vi "TestExecutive V2.vi"() -> ()   [LabVIEW 2025]
uses:
  controls/TestDefinition.ctl
  controls/SingleTest.ctl
  controls/TestType.ctl
  controls/HTR Test Options.ctl
  controls/TestFailOptions.ctl
  controls/TED4015 Status.ctl
  controls/Diode Test Options.ctl
  <vilib>/addons/_JKI Toolkits/State Machine/_JKI_lib_State_Machine.llb/Periodic Trigger__ogtk__JKI-SM__jki_lib_state_machine.vi
  <vilib>/addons/_JKI Toolkits/State Machine/_JKI_lib_State_Machine.llb/Select State(s)_err__jki_lib_state_machine.vi
  <userlib>/_OpenG.lib/time/time.llb/openg_time.lvlib
panel:
  in  "Exit":bool
  out "Camera":string="HD Pro Webcam C920"
  out "TopFolderPath":path=path "d:/LTM Tests/MechanismLTM/HeaterTest_25-11-11_16-31-07"
  out "TopFolderPrefix":string="HeaterTest_25-11-11_16-31-07"
  out "Status":string="Setup - Fill in fields and press Next to Continue"
  in  "Main Tabs":T1(tab)
  in  "Cycles To Run":i32=1 min=1 max=200
  in  "Next1":bool
  in  "Loggers Directory":path=path "d:/LTM Tests/MechanismLTM"
  in  "Test Name":string="HeaterTest"
  in  "FFMPEG exe":path=path "C:/Program Files/FFMpeg/bin/ffmpeg.exe"
  in  "Path to Actuation Script":path=path "C:/Users/dpl/Documents/ob_egse/src/main.py"
  in  "StartCycle":i32
  in  "Tab Control":T2(tab)=enum."Diodes"
  in  "TVC_Temperatures":waveform(dbl)[](array[waveform])=[{"t0"=timestamp(3820413812.1049423 s since 1904-01-01), "dt"=1.0, "Y"=[-45.0], "attributes"=variant("NI_ChannelName"=variant(string "3A"))}, {"t0"=timestamp(3820413812.1049423 s since 1904-01-01), "dt"=1.0, "Y"=[0.1969585335155295], "attributes"=variant("NI_ChannelName"=variant(string "3B"))}, {"t0"=timestamp(3820413812.1049423 s since 1904-01-01), "dt"=1.0, "Y"=[0.2898606356704896], "attributes"=variant("NI_ChannelName"=variant(string "3C"))}, {"t0"=timestamp(3820413812.1049423 s since 1904-01-01), "dt"=1.0, "Y"=[0.3274623555028864], "attributes"=variant("NI_ChannelName"=variant(string "3D"))}, {"t0"=timestamp(3820413812.1049423 s since 1904-01-01), "dt"=1.0, "Y"=[0.3794250746071903], "attributes"=variant("NI_ChannelName"=variant(string "4A"))}, {"t0"=timestamp(3820413812.1049423 s since 1904-01-01), "dt"=1.0, "Y"=[0.7650917242886434], "attributes"=variant("NI_ChannelName"=variant(string "4B"))}, {"t0"=timestamp(3820413812.1049423 s since 1904-01-01), "dt"=1.0, "Y"=[0.4416685188806395], "attributes"=variant("NI_ChannelName"=variant(string "4C"))}, {"t0"=timestamp(3820413812.1049423 s since 1904-01-01), "dt"=1.0, "Y"=[0.7497510727682433], "attributes"=variant("NI_ChannelName"=variant(string "4D"))}, {"t0"=timestamp(3820413812.1049423 s since 1904-01-01), "dt"=1.0, "Y"=[0.8015992709050663], "attributes"=variant("NI_ChannelName"=variant(string "Target"))}]
  out "ChannelNames":string[](array[string])=["3A", "3B", "3C", "3D", "4A", "4B", "4C", "4D", "Target"]
  in  "ControlChannel":u16(ring) items=["3A", "3B", "3C", "3D", "4A", "4B", "4C", "4D", "Target"]
  in  "TLUP_Temperatures":waveform(dbl)[](array[waveform])=[{"t0"=timestamp(3820413812.102944 s since 1904-01-01), "dt"=1.0, "Y"=[23.56152], "attributes"=variant("NI_ChannelName"=variant(string "TLUP_0"))}, {"t0"=timestamp(3820413812.102944 s since 1904-01-01), "dt"=1.0, "Y"=[-999.0], "attributes"=variant("NI_ChannelName"=variant(string "TLUP_1"))}, {"t0"=timestamp(3820413812.102944 s since 1904-01-01), "dt"=1.0, "Y"=[-999.0], "attributes"=variant("NI_ChannelName"=variant(string "TLUP_2"))}, {"t0"=timestamp(3820413812.102944 s since 1904-01-01), "dt"=1.0, "Y"=[-999.0], "attributes"=variant("NI_ChannelName"=variant(string "TLUP_3"))}, {"t0"=timestamp(3820413812.102944 s since 1904-01-01), "dt"=1.0, "Y"=[nan], "attributes"=variant("NI_ChannelName"=variant(string "TLUP_4"))}, {"t0"=timestamp(3820413812.102944 s since 1904-01-01), "dt"=1.0, "Y"=[nan], "attributes"=variant("NI_ChannelName"=variant(string "TLUP_5"))}, {"t0"=timestamp(3820413812.102944 s since 1904-01-01), "dt"=1.0, "Y"=[nan], "attributes"=variant("NI_ChannelName"=variant(string "TLUP_6"))}, {"t0"=timestamp(3820413812.102944 s since 1904-01-01), "dt"=1.0, "Y"=[nan], "attributes"=variant("NI_ChannelName"=variant(string "TLUP_7"))}]
  in  "PSU_Monitor":waveform(dbl)[](array[waveform])=[{"t0"=timestamp(3820413812.1099424 s since 1904-01-01), "dt"=1.0, "Y"=[2.52], "attributes"=variant("NI_ChannelName"=variant(string "Board_Voltage_0"))}, {"t0"=timestamp(3820413812.1153584 s since 1904-01-01), "dt"=1.0, "Y"=[-0.009], "attributes"=variant("NI_ChannelName"=variant(string "Board_Voltage_0"))}, {"t0"=timestamp(3820413812.1099424 s since 1904-01-01), "dt"=1.0, "Y"=[-0.017], "attributes"=variant("NI_ChannelName"=variant(string "Board_Current_0"))}, {"t0"=timestamp(3820413812.1153584 s since 1904-01-01), "dt"=1.0, "Y"=[0.0], "attributes"=variant("NI_ChannelName"=variant(string "Board_Current_0"))}]
  in  "PSU Enable":bool
  in  "Heater Monitor":waveform(dbl)[](array[waveform])=[{"t0"=timestamp(3820413812.092942 s since 1904-01-01), "dt"=1.0, "Y"=[-0.005], "attributes"=variant("NI_ChannelName"=variant(string "Heater_Voltage"))}, {"t0"=timestamp(3820413812.092942 s since 1904-01-01), "dt"=1.0, "Y"=[1.55], "attributes"=variant("NI_ChannelName"=variant(string "Heater_Current"))}]
  in  "Heater Enable":bool
  in  "COM Port":i32=21 min=1 max=63 step=1
  in  "Video Camera":u16(ring) items=["USB Camera"]
  in  "TED":waveform(dbl)[](graph)
  in  "TEC On":bool[](array[boolean])=[FALSE, FALSE]
  in  "TED Status":T3[](array[typedef])=[{"Output"=TRUE, "SetPoint"=0.0, "Temperature"=0.0, "Current"=0.0, "Voltage"=0.0, "CableTrip"=FALSE, "TransducerTrip"=FALSE, "OverTemp"=FALSE}, {"Output"=TRUE, "SetPoint"=0.0, "Temperature"=0.0, "Current"=0.0, "Voltage"=0.0, "CableTrip"=FALSE, "TransducerTrip"=FALSE, "OverTemp"=FALSE}]
  in  "LED_Stimulate":bool
  in  "LED_Illuminate":bool
  in  "Diode Currents":waveform(dbl)[](graph)=[{"t0"=timestamp(0 s since 1904-01-01), "dt"=1.0, "Y"=[2.0]}, {"t0"=timestamp(0 s since 1904-01-01), "dt"=1.0, "Y"=[2.0]}]
  in  "Next2":bool
  in  "Server IP":u16(ring) items=["localhost", "172.17.52.10"]
  in  "SaveTests":bool
  in  "TestDefinition":T4={"Tests"=[{"TTrigger"=-130.0, "Direction"=enum."Falling", "TDelay"=0.0, "Type"=enum."No Test", "Pre-Log (s)"=0.0, "Duration (s)"=0.0, "Post-Log(s)"=0.0}, {"TTrigger"=-80.0, "Direction"=enum."Rising", "TDelay"=0.0, "Type"=enum."Heater Test", "Pre-Log (s)"=10.0, "Duration (s)"=10.0, "Post-Log(s)"=2.0}, {"TTrigger"=-50.0, "Direction"=enum."Rising", "TDelay"=0.0, "Type"=enum."Diode Test", "Pre-Log (s)"=20.0, "Duration (s)"=20.0, "Post-Log(s)"=20.0}, {"TTrigger"=-45.0, "Direction"=enum."Rising", "TDelay"=0.0, "Type"=enum."Actuation Test", "Pre-Log (s)"=10.0, "Duration (s)"=20.0, "Post-Log(s)"=10.0}, {"TTrigger"=30.0, "Direction"=enum."Rising", "TDelay"=0.0, "Type"=enum."Actuation Test", "Pre-Log (s)"=10.0, "Duration (s)"=30.0, "Post-Log(s)"=100.0}, {"TTrigger"=40.0, "Direction"=enum."Rising", "TDelay"=30.0, "Type"=enum."No Test", "Pre-Log (s)"=10.0, "Duration (s)"=30.0, "Post-Log(s)"=100.0}], "ActuationsPerLoop"=2, "Temperature Log Period(ms)"=1000, "PSU  Log Period (ms)"=100} {"Tests"."Post-Log(s)" format="%#_13g"; "Tests"."Pre-Log (s)" format="%#_13g"; "Tests"."Duration (s)" format="%#_13g"}
  in  "Next Button 3":bool
  in  "Heater Test Options":T7={"Heater Nominal Current (A)"=0.67, "Heater Current Tolerance (%)"=20.0, "Fail Text"="", "Fail Option"=enum."Ignore"} {"Heater Current Tolerance (%)" min=1.0 max=100.0; "Heater Nominal Current (A)" min=0.0 max=1.0}
  in  "Diode Test Options":T9={"Temp.Tol"=0.1, "Max IDark"=[], "Min ILight"=[0.1, 1e-08]}
  out "Messages":string
  out "ACT Fault":bool
  out "TVC_StopAfterCycle":bool
  out "Diode Logging":bool
  out "Master Logging":bool
  out "DelayRemaining":string
  out "HTR On":bool
  out "Temperatures":dynamicdata(graph)=[{"t0"=timestamp(3820413812.1049423 s since 1904-01-01), "dt"=1.0, "Y"=[-45.0], "attributes"=variant("NI_ChannelName"=variant(string "3A"))}, {"t0"=timestamp(3820413812.1049423 s since 1904-01-01), "dt"=1.0, "Y"=[0.1969585335155295], "attributes"=variant("NI_ChannelName"=variant(string "3B"))}, {"t0"=timestamp(3820413812.1049423 s since 1904-01-01), "dt"=1.0, "Y"=[0.2898606356704896], "attributes"=variant("NI_ChannelName"=variant(string "3C"))}, {"t0"=timestamp(3820413812.1049423 s since 1904-01-01), "dt"=1.0, "Y"=[0.3274623555028864], "attributes"=variant("NI_ChannelName"=variant(string "3D"))}, {"t0"=timestamp(3820413812.1049423 s since 1904-01-01), "dt"=1.0, "Y"=[0.3794250746071903], "attributes"=variant("NI_ChannelName"=variant(string "4A"))}, {"t0"=timestamp(3820413812.1049423 s since 1904-01-01), "dt"=1.0, "Y"=[0.7650917242886434], "attributes"=variant("NI_ChannelName"=variant(string "4B"))}, {"t0"=timestamp(3820413812.1049423 s since 1904-01-01), "dt"=1.0, "Y"=[0.4416685188806395], "attributes"=variant("NI_ChannelName"=variant(string "4C"))}, {"t0"=timestamp(3820413812.1049423 s since 1904-01-01), "dt"=1.0, "Y"=[0.7497510727682433], "attributes"=variant("NI_ChannelName"=variant(string "4D"))}, {"t0"=timestamp(3820413812.1049423 s since 1904-01-01), "dt"=1.0, "Y"=[0.8015992709050663], "attributes"=variant("NI_ChannelName"=variant(string "Target"))}, {"t0"=timestamp(3820413812.102944 s since 1904-01-01), "dt"=1.0, "Y"=[23.56152], "attributes"=variant("NI_ChannelName"=variant(string "TLUP_0"))}, {"t0"=timestamp(3820413812.102944 s since 1904-01-01), "dt"=1.0, "Y"=[-999.0], "attributes"=variant("NI_ChannelName"=variant(string "TLUP_1"))}, {"t0"=timestamp(3820413812.102944 s since 1904-01-01), "dt"=1.0, "Y"=[-999.0], "attributes"=variant("NI_ChannelName"=variant(string "TLUP_2"))}, {"t0"=timestamp(3820413812.102944 s since 1904-01-01), "dt"=1.0, "Y"=[-999.0], "attributes"=variant("NI_ChannelName"=variant(string "TLUP_3"))}, {"t0"=timestamp(3820413812.102944 s since 1904-01-01), "dt"=1.0, "Y"=[nan], "attributes"=variant("NI_ChannelName"=variant(string "TLUP_4"))}, {"t0"=timestamp(3820413812.102944 s since 1904-01-01), "dt"=1.0, "Y"=[nan], "attributes"=variant("NI_ChannelName"=variant(string "TLUP_5"))}, {"t0"=timestamp(3820413812.102944 s since 1904-01-01), "dt"=1.0, "Y"=[nan], "attributes"=variant("NI_ChannelName"=variant(string "TLUP_6"))}, {"t0"=timestamp(3820413812.102944 s since 1904-01-01), "dt"=1.0, "Y"=[nan], "attributes"=variant("NI_ChannelName"=variant(string "TLUP_7"))}]
  out "Trigger Point Reading":dbl=-45.0
  out "ACT Logging":bool
  out "HTR Log":bool
  out "TVC_CyclesRemaining":i32
  in  "TVC_CycleNumber":i32
  out "HTR_Fault":bool
  out "TEC Fault":bool
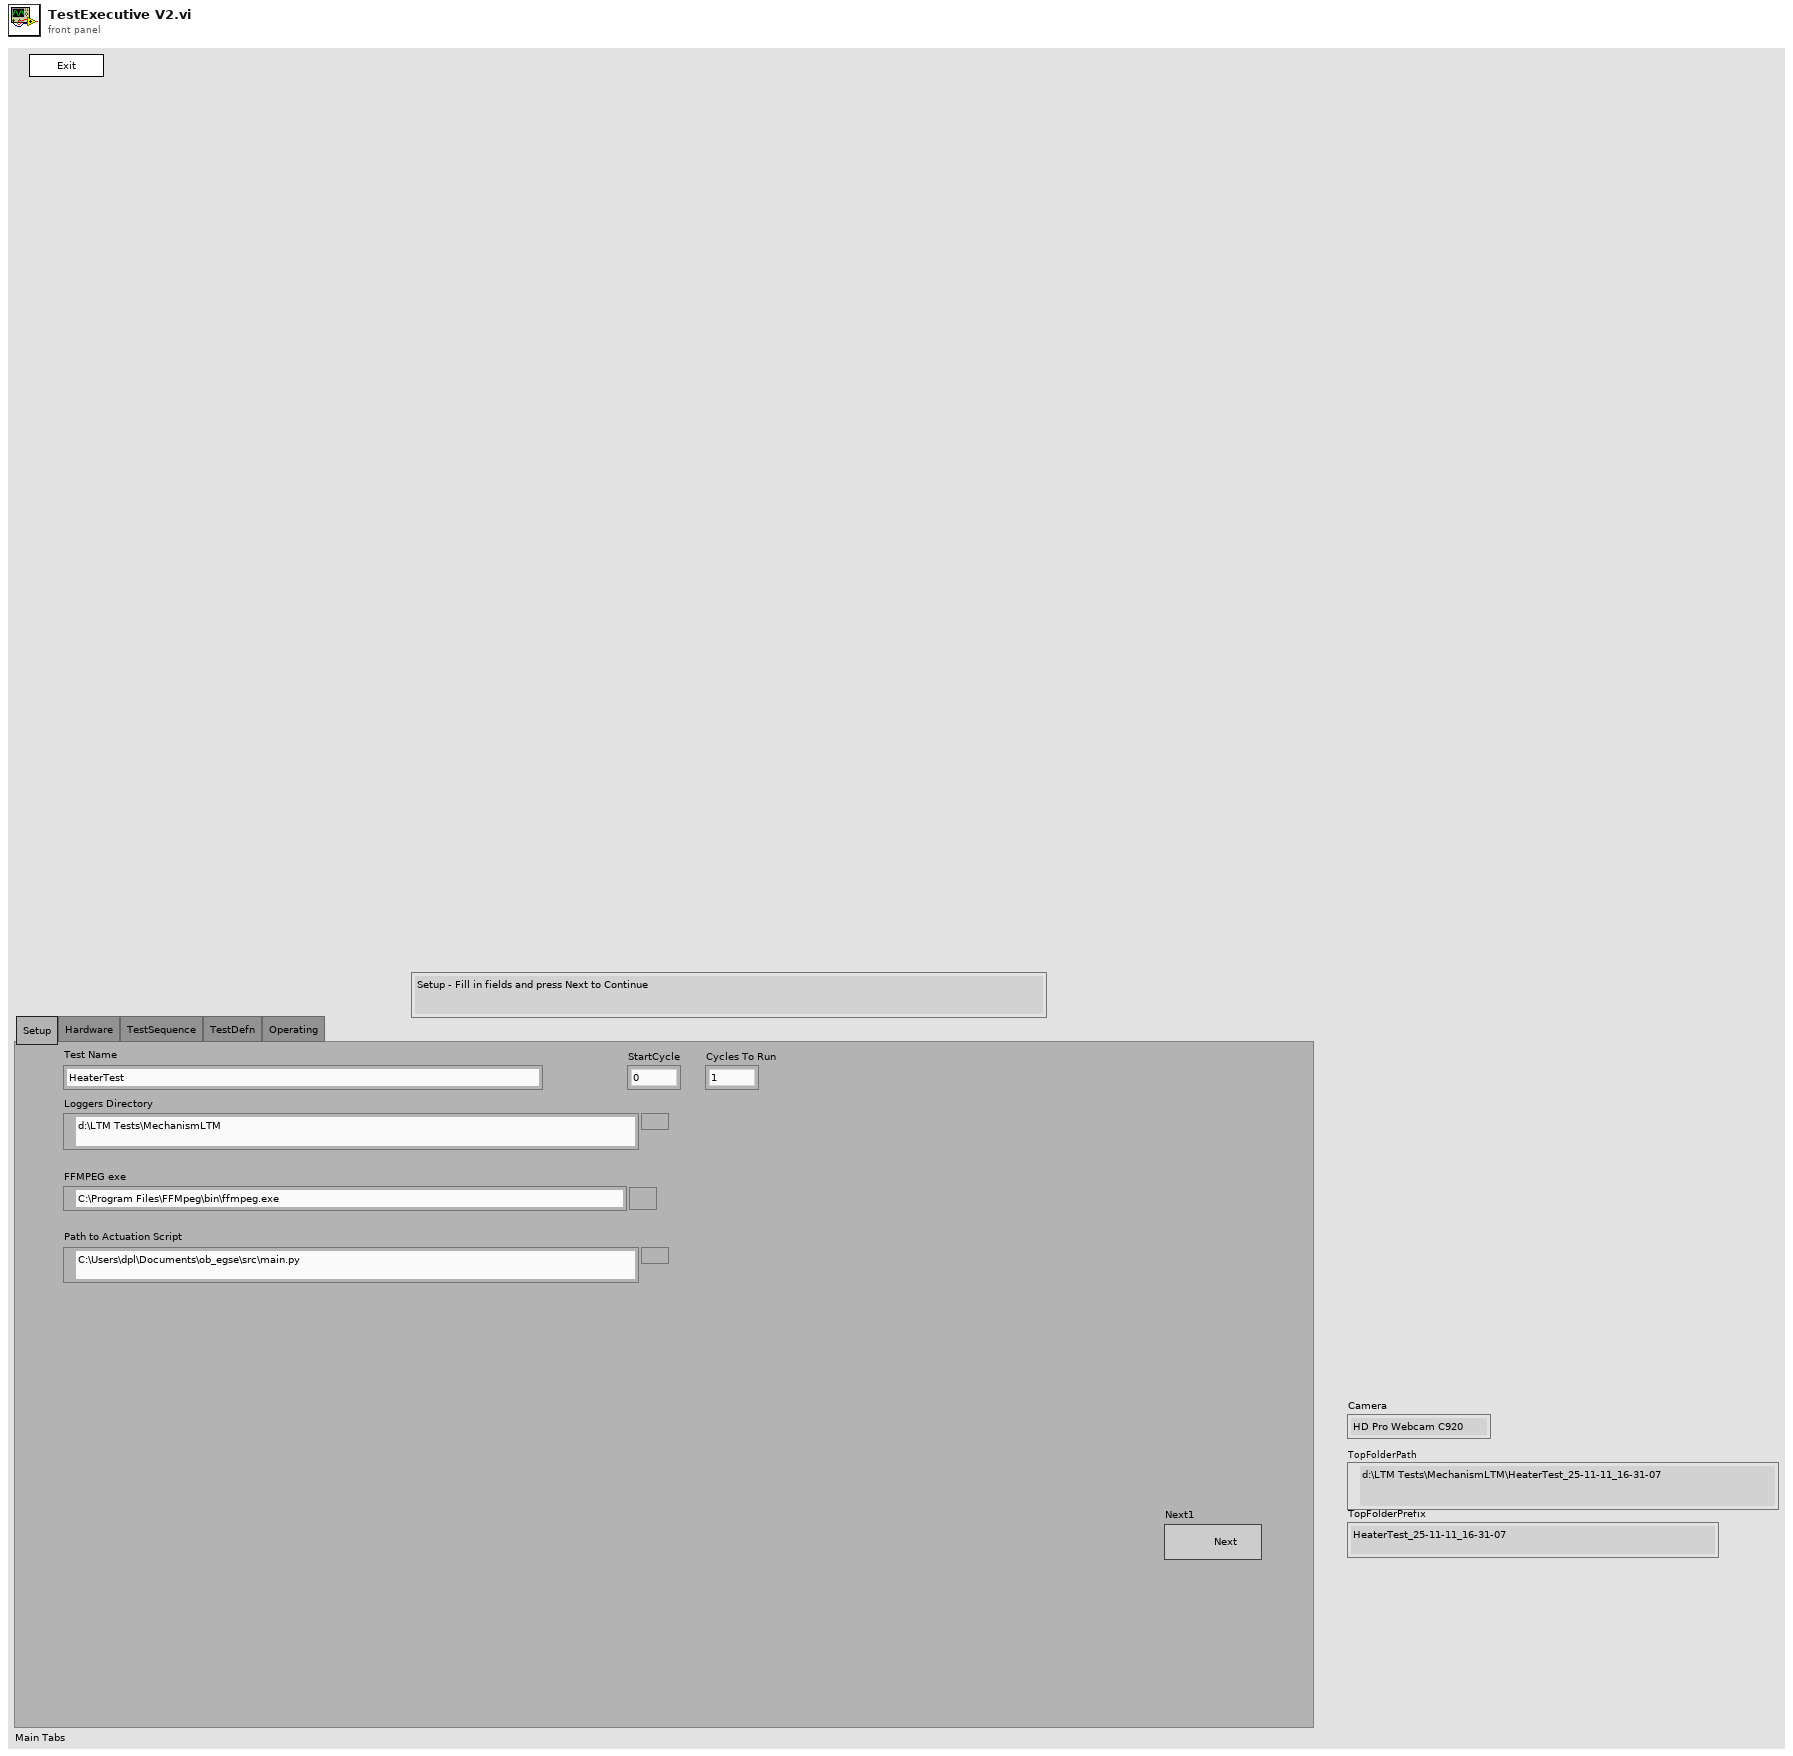
[diagram p1: front panel]
types:
  T1 = enum32{"Setup", "Hardware", "TestSequence", "TestDefn", "Operating"}
  T2 = enum32{"Temperatures", "PSUs", "TED4015s", "Diodes"}
  T3 = typedef "TED4015 Status.ctl" = cluster{"Output":bool, "SetPoint":dbl, "Temperature":dbl, "Current":dbl, "Voltage":dbl, "CableTrip":bool, "TransducerTrip":bool, "OverTemp":bool}
  T4 = typedef "TestDefinition.ctl" = cluster{"Tests":T5[], "ActuationsPerLoop":i32, "Temperature Log Period(ms)":i64, "PSU  Log Period (ms)":i64}
  T5 = typedef "SingleTest.ctl" = cluster{"TTrigger":dbl, "Direction":enum16{"Rising", "Falling"}, "TDelay":dbl, "Type":T6, "Pre-Log (s)":dbl, "Duration (s)":dbl, "Post-Log(s)":dbl}
  T6 = typedef "TestType.ctl" = enum16{"No Test", "Heater Test", "Actuation Test", "Diode Test"}
  T7 = typedef "HTR Test Options.ctl" = cluster{"Heater Nominal Current (A)":dbl, "Heater Current Tolerance (%)":dbl, "Fail Text":string, "Fail Option":T8}
  T8 = typedef "TestFailOptions.ctl" = enum16{"Ignore", "Halt End Cycle", "Skip Rest Of Cycle"}
  T9 = typedef "Diode Test Options.ctl" = cluster{"Temp.Tol":dbl, "Max IDark":dbl[], "Min ILight":dbl[]}
  T10 = enum32{"Invalid", "Standard", "Closed", "Hidden", "Minimized", "Maximized"}
  T11 = enum32{"invalid app kind", "Development System", "Run Time System", "Student Edition", "Embedded LabVIEW", "Evaluation", "Custom"}
  T12 = enum32{"Invalid Status", "Unconnected", "Active", "Idle", "Error", "Connecting"}
  T13 = cluster{"Core":cluster{"Current VI Reference":refnum<vi>, "Close Panel on Exit?":bool}, "CurrentCycle":i32, "TestNumber":i32, "TopFolderPath":path, "LogFilePath":path, "TestPrefix":string, "CurrentTest":T5}
  T14 = cluster{"Current VI Reference":refnum<vi>, "Close Panel on Exit?":bool}
  T15 = typedef "LVDataSocketStatusTypeDef.ctl" = cluster{"Code":enum32{"Invalid Status", "Unconnected", "Active", "Idle", "Error", "Connecting"}, "Text":string}
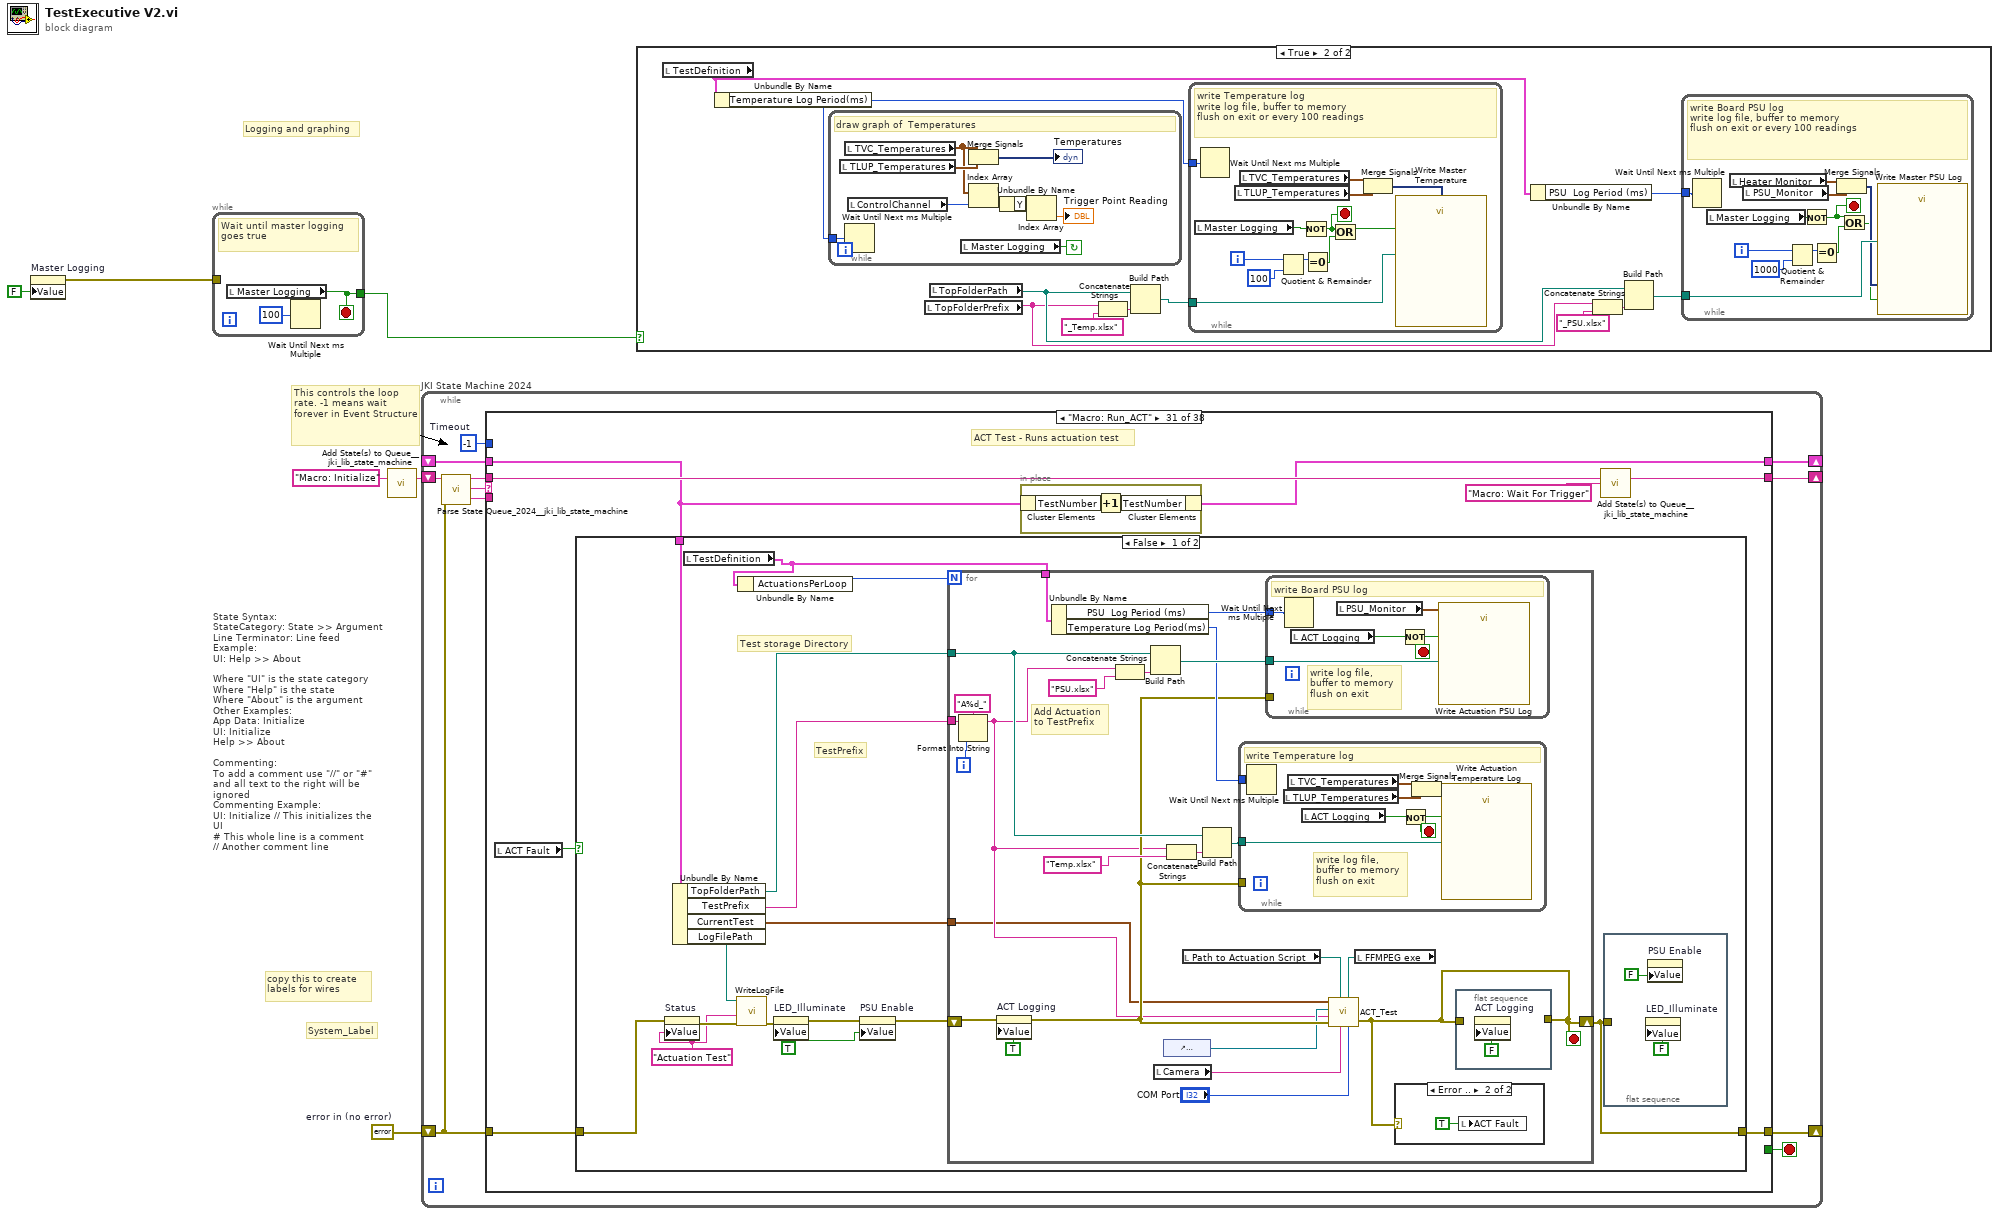
[diagram p0: block diagram]
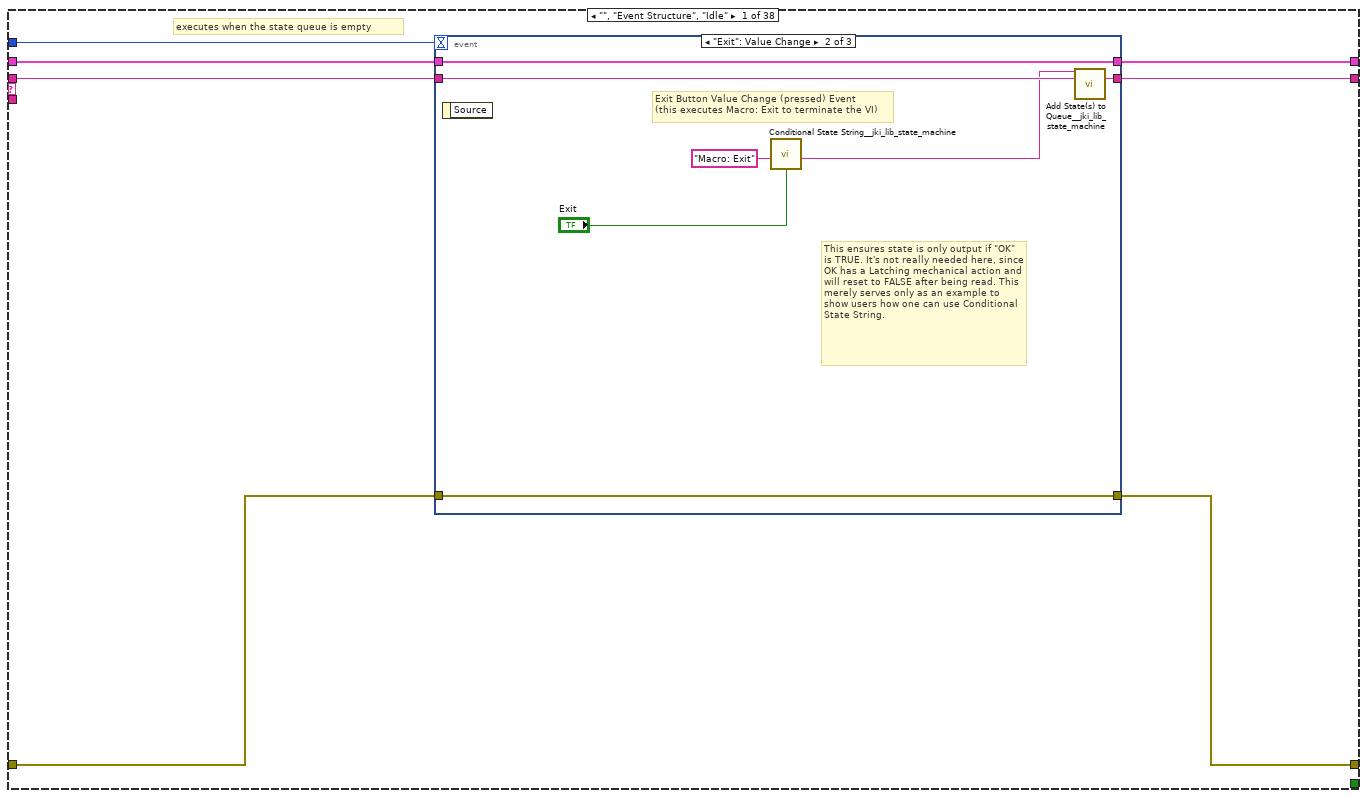
[diagram p2: hidden frame]
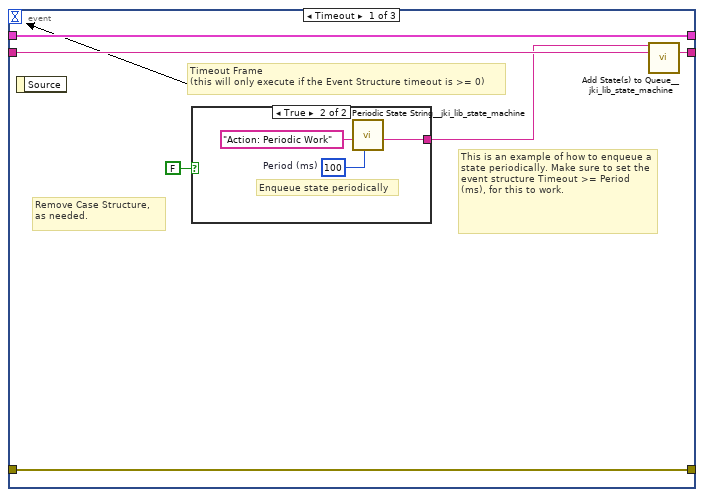
[diagram p3: hidden frame]
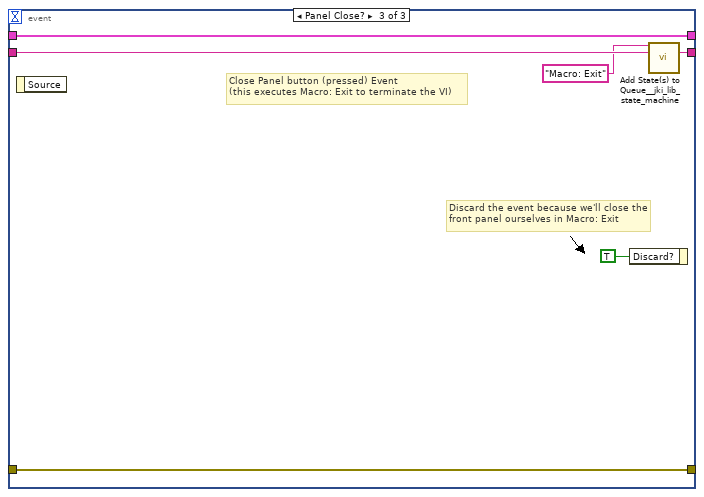
[diagram p5: hidden frame]
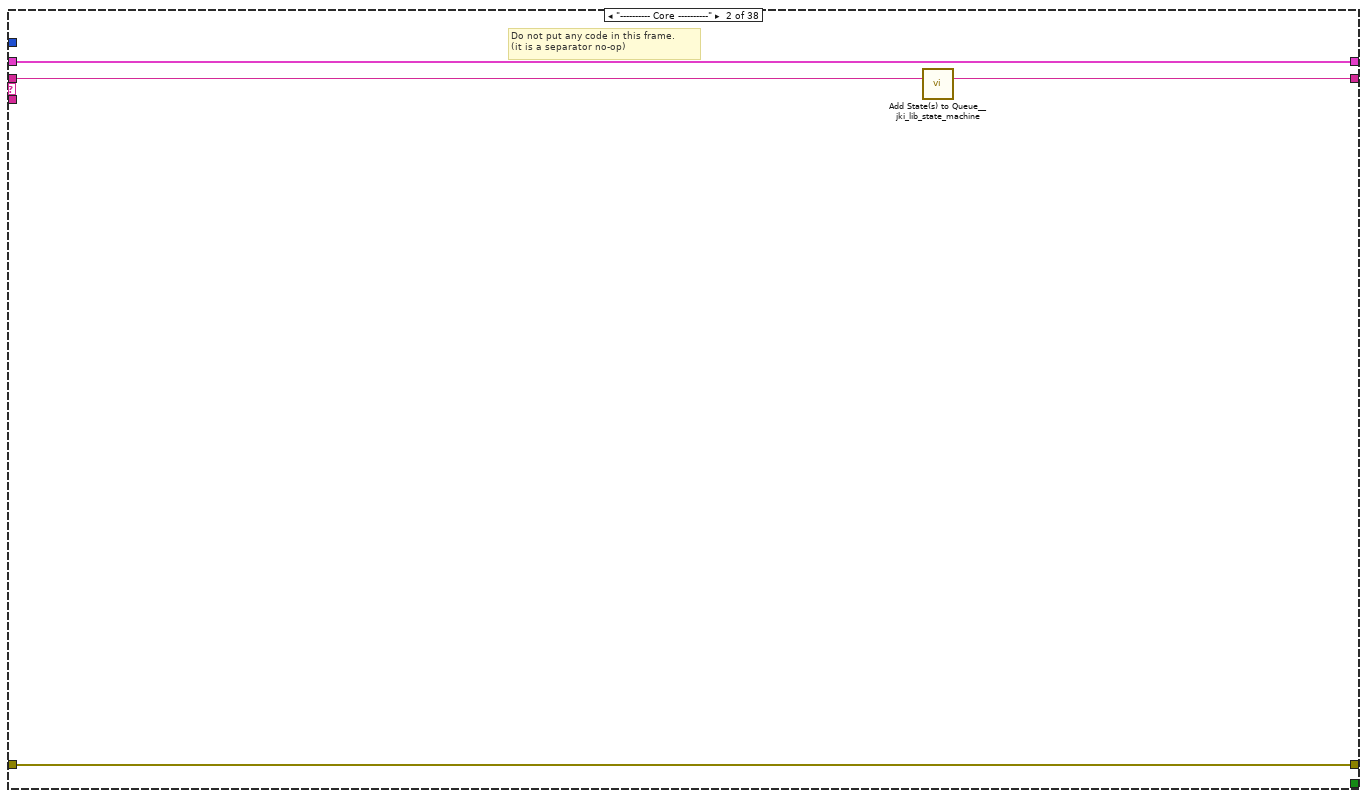
[diagram p6: hidden frame]
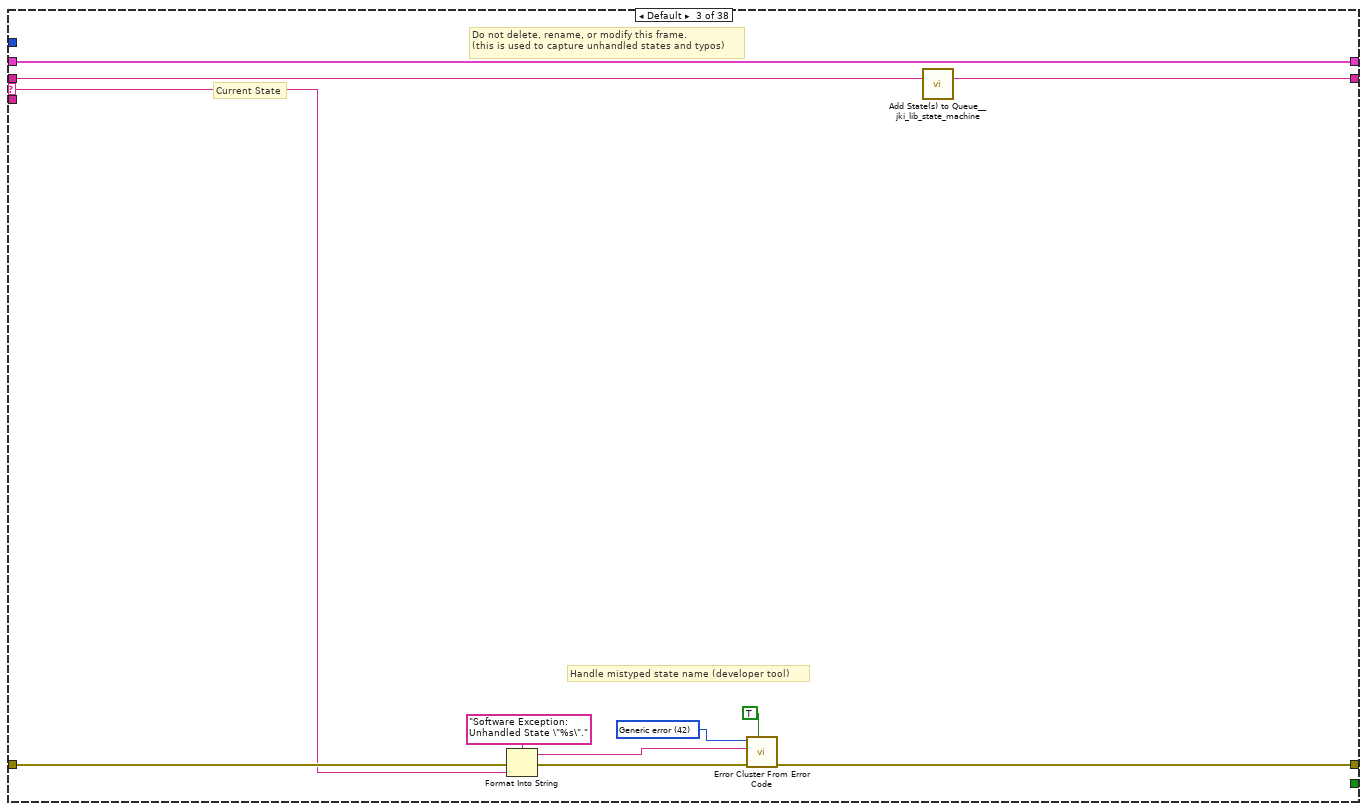
[diagram p7: hidden frame]
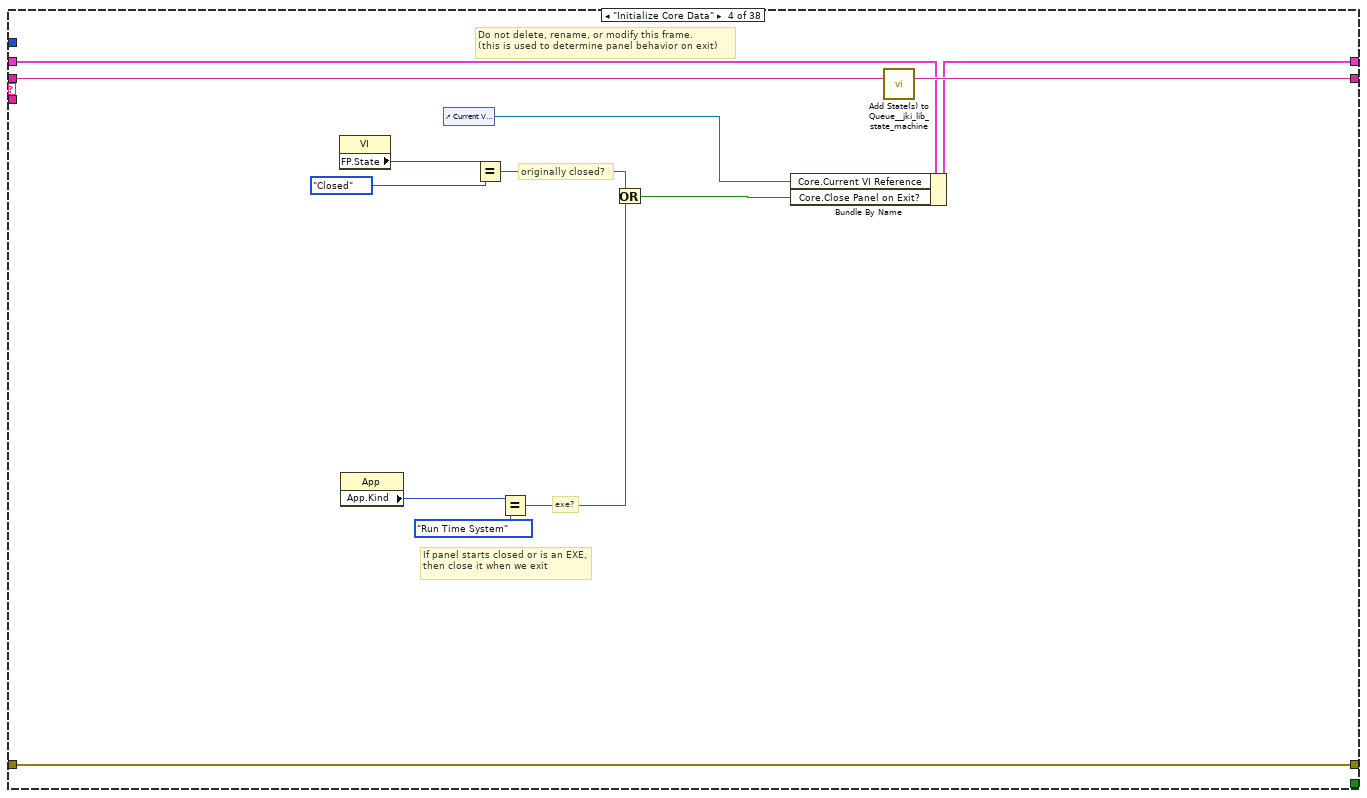
[diagram p8: hidden frame]
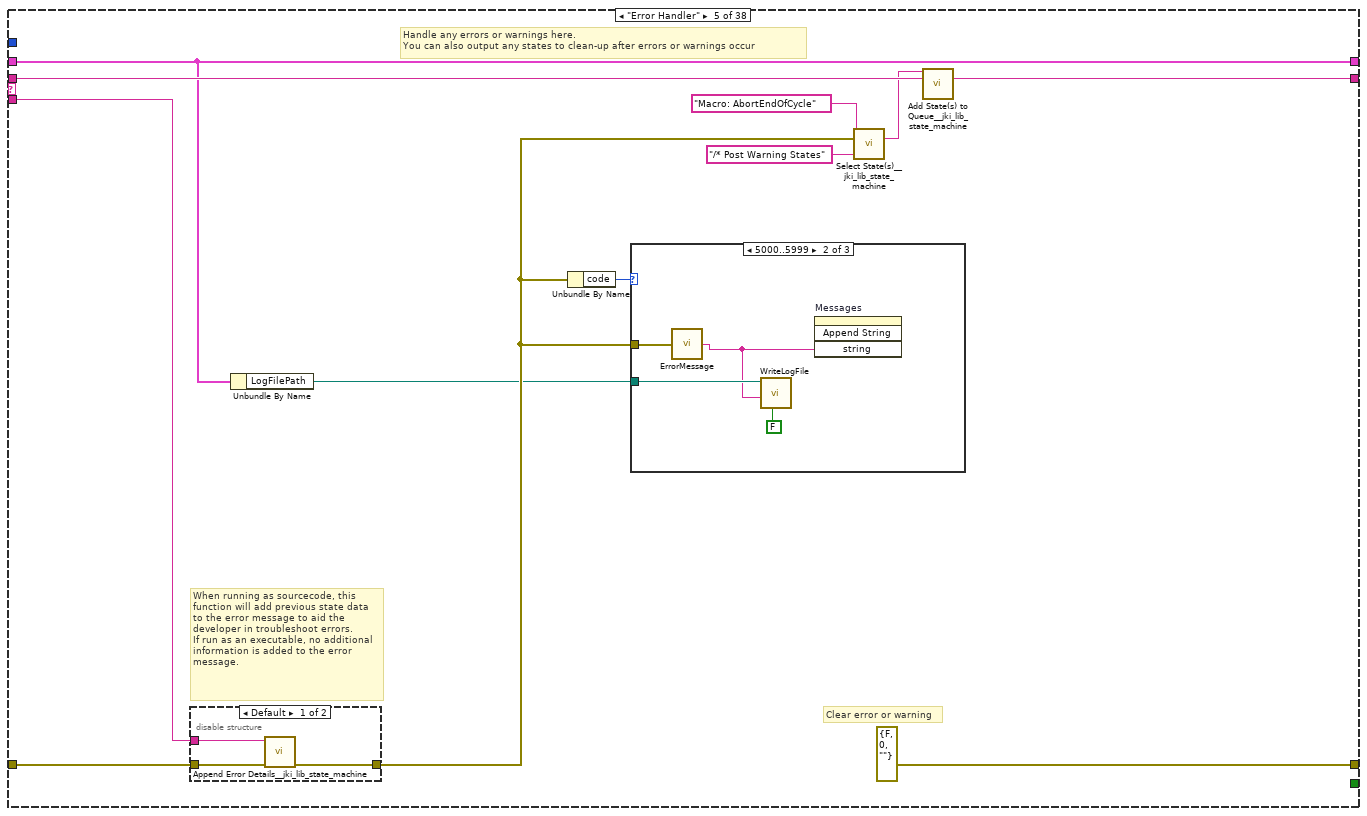
[diagram p9: hidden frame]
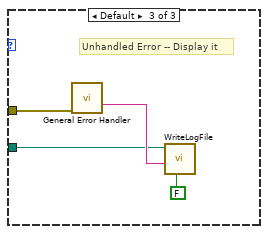
[diagram p11: hidden frame]
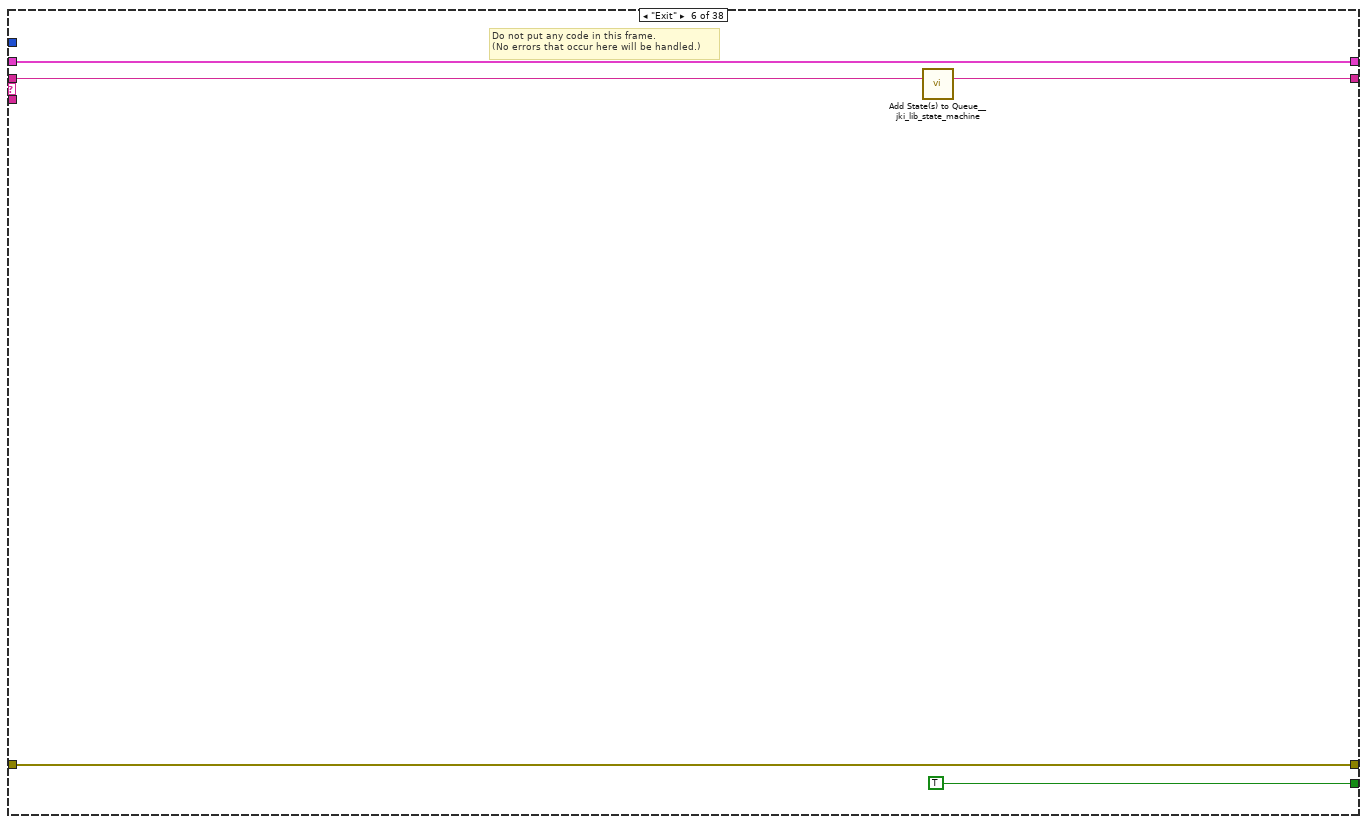
[diagram p13: hidden frame]
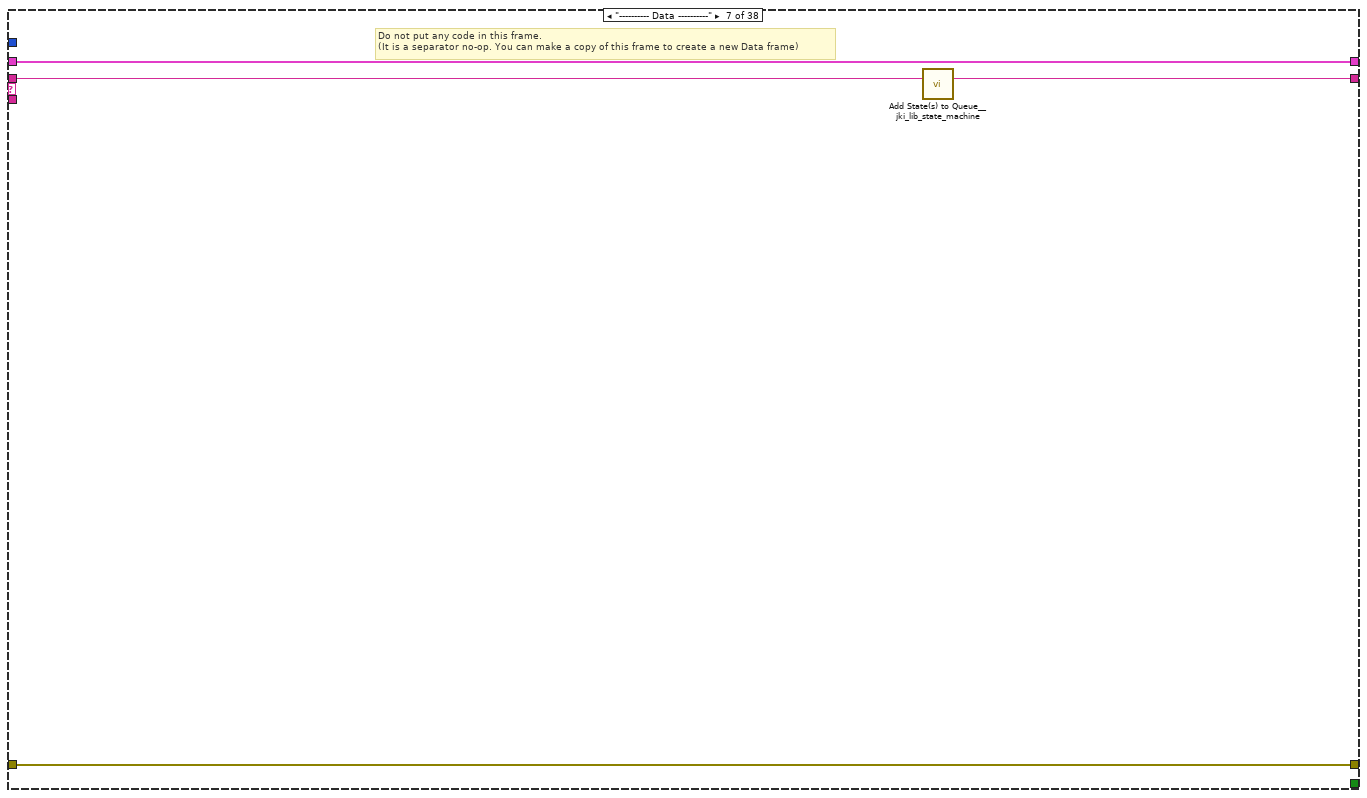
[diagram p14: hidden frame]
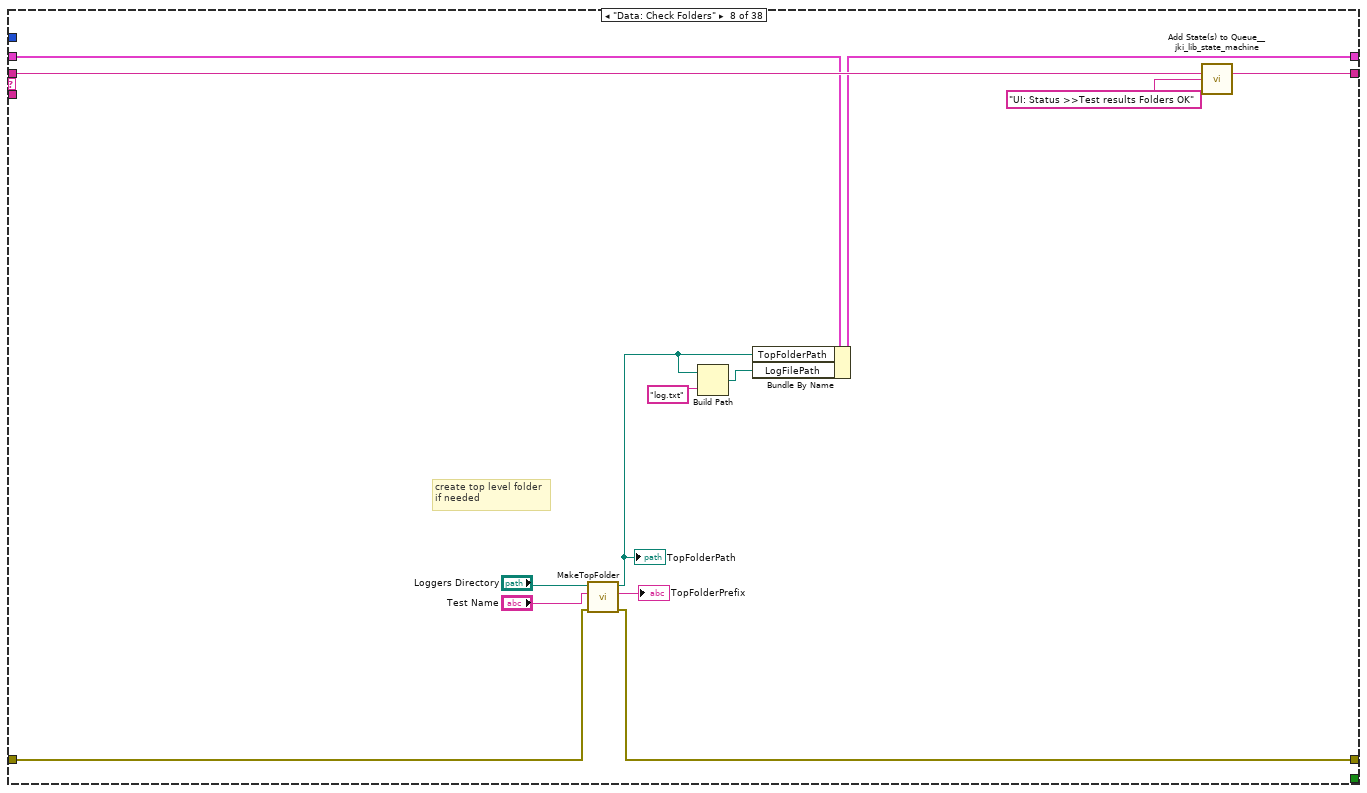
[diagram p15: hidden frame]
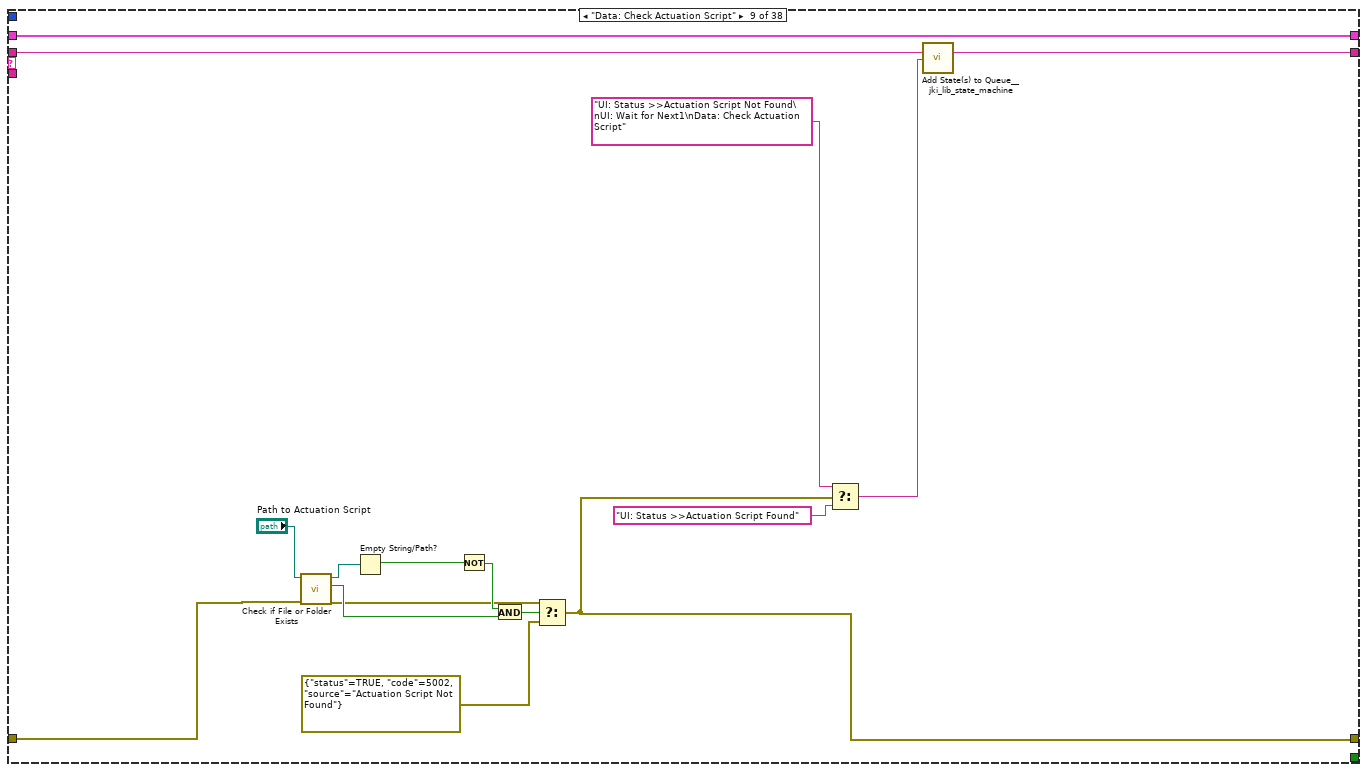
[diagram p16: hidden frame]
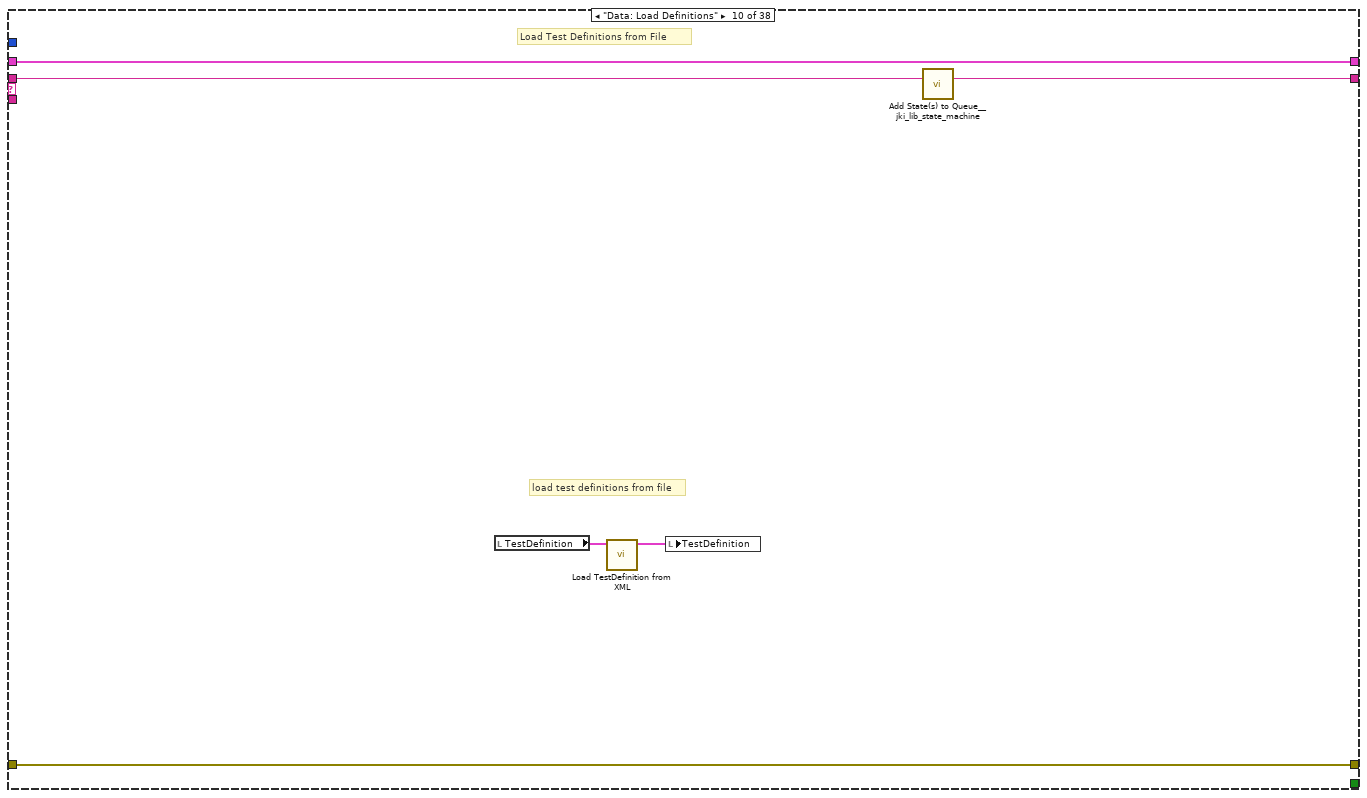
[diagram p17: hidden frame]
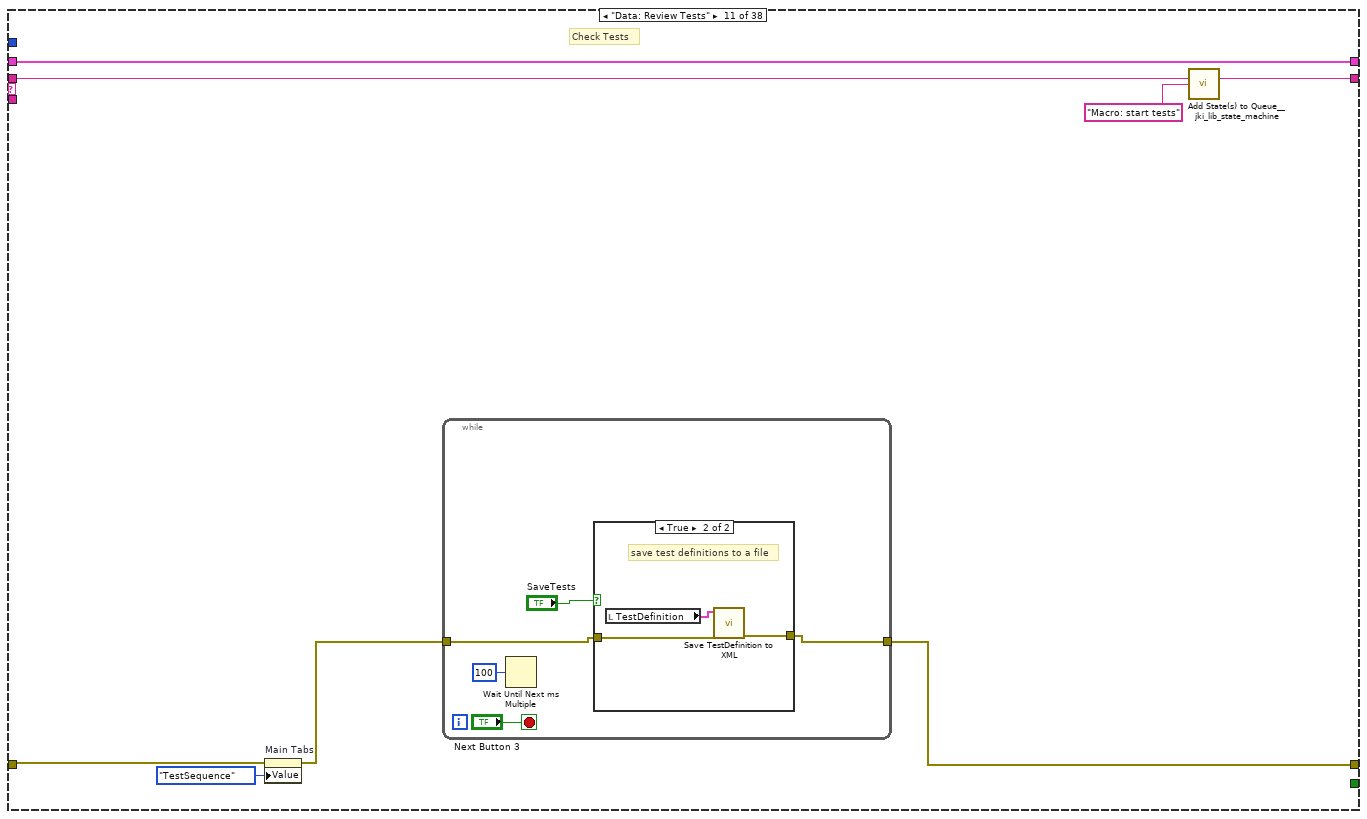
[diagram p18: hidden frame]
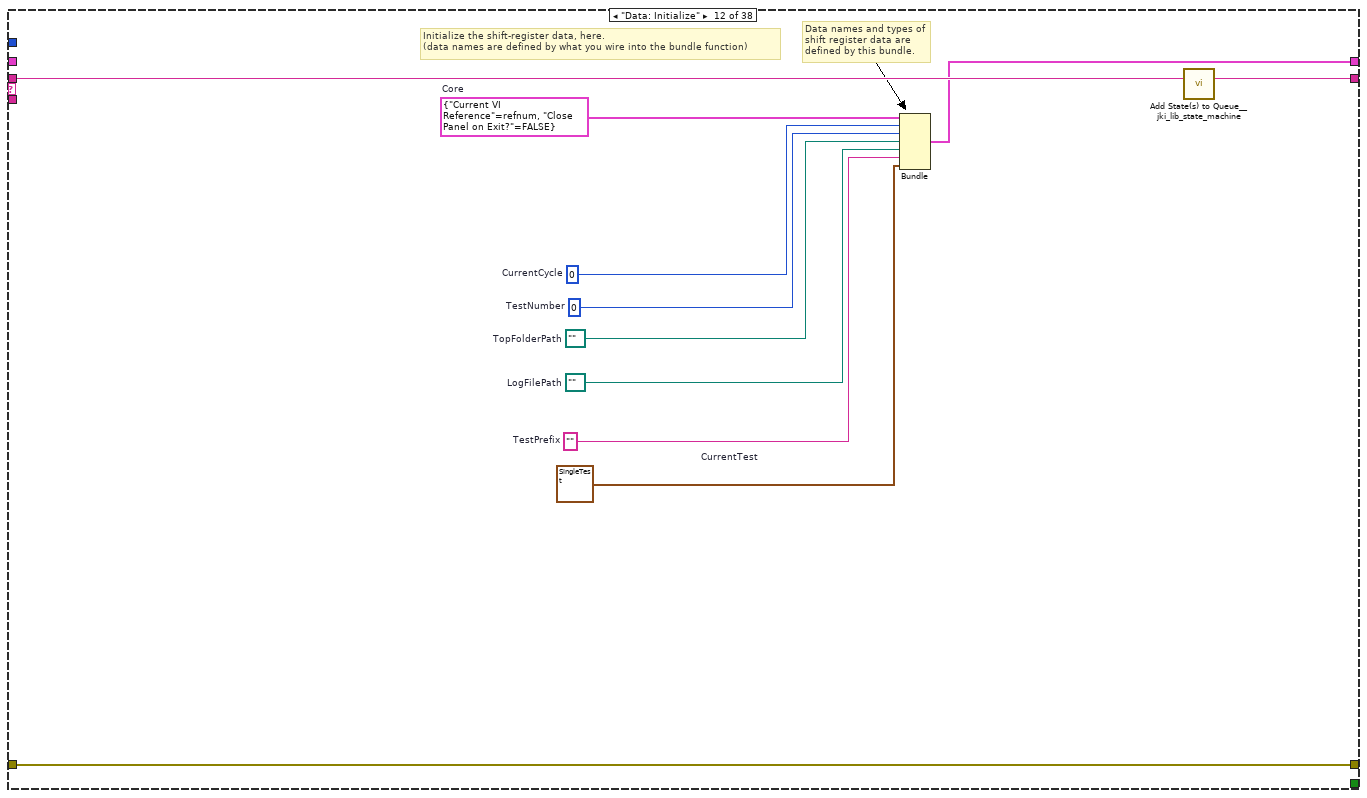
[diagram p20: hidden frame]
diagram:
  w1 = errorcluster {"status"=FALSE, "code"=0, "source"=""}  # error in (no error)
  # "State Syntax:\nStateCategory: State >> Argument\nLine Terminator: Line feed\nExample:\nUI: Help >> About\n\nWhere \"UI\" is the state category\nWhere \"Help\" is the state\nWhere \"About\" is the argument\nOther Examples:\nApp Data: Initialize\nUI: Initialize\nHelp >> About\n\nCommenting:\nTo add a comment use \"//\" or \"#\" and all text to the right will be ignored\nCommenting Example:\nUI: Initialize // This initializes the UI\n# This whole line is a comment\n// Another comment line"
  # "copy this to create labels for wires"
  # "This controls the loop rate. -1 means wait forever in Event Structure"
  # "System_Label"
  # "Logging and graphing"
  n1 = property on="Master Logging" class="Bool (strict)"("Value"=FALSE ("Master Logging")) -> (error out=w6:errorcluster)  [unwired: 2 in, 1 out]
  n2 = while {
    tunnel: [w7] -> w4
    tunnel: w6 -> [_]
    stop <- w7 stop-if-true
    # "Wait until master logging goes true"
    n3 = local read "Master Logging"() -> (w7:bool)
    n4 = Wait Until Next ms Multiple(millisecond multiple=u32 100) -> ()  [unwired: 1 out]
  }
  n5 = call <vilib>:"Add State(s) to Queue__jki_lib_state_machine.vi"("State(s) in (\"\")"="Macro: Initialize") -> ("States Out"=w3:string)  [unwired: 14 in]
  n6 = while "JKI State Machine 2024" {
    shift-right: [w12] -> _
    shift-left: _ -> [w11]
    shift-right: [w15] -> _
    shift-left: w1 -> [w9]
    shift-right: [w14] -> _
    shift-left: w3 -> [w16]
    stop <- w13 stop-if-true
    w10 = -1  # Timeout
    n7 = call <vilib>:"Parse State Queue_2024__jki_lib_state_machine.vi"("State Queue"=w16, "Error In (no error)"=w9) -> ("Remaining States"=w18:string, "Current State"=w19:string, "Arguments"=w17:string)  [unwired: 11 in]
    n8 = case shown="\"Macro: Run_ACT\"" w19 {
      selector: w19 -> [_ _ w53 _ _ _ _ _ _ _ _ _ _ _ _ _ _ _ _ _ _ _ _ _ _ _ _ _ _ _ _ _ _ _ _ _ _ _]
      tunnel: w18 -> [w26 w52 w57 w76 w88 w105 w109 w122 w138 w144 w152 w172 w178 w182 w186 w196 w203 w209 w228 w246 w257 w326 w331 w344 w359 w371 w423 w459 w469 w528 w593 w662 w679 w688 w692 w701 w726 w735]
      tunnel: w17 -> [_ _ _ _ w84 _ _ _ _ _ _ _ _ _ _ _ _ w204 _ w241 w251 _ _ w336 _ _ _ _ _ _ _ _ _ _ _ _ _ _]
      tunnel: w11 -> [w24 w49 w55 w69 w78 w103 w106 w120 w136 w141 w150 _ w173 w179 w183 w194 w201 w207 w226 w244 w253 w323 w328 w342 w357 w361 w421 w456 w465 w523 w589 w655 w674 w686 w689 w699 w724 w733]
      tunnel: [w23 w50 w59 w73 errorcluster {"status"=FALSE, "code"=0, "source"=""} ("error out") w102 w107 w115 w126 w142 w147 w169 w174 w180 w184 w193 w197 w205 w213 w242 w254 w324 w329 w337 w351 w368 w411 w457 w464 w522 w587 w657 w676 w683 w690 w693 w715 w728] -> w15
      tunnel: w9 -> [w20 w50 w58 w73 w85 w102 w107 w116 w128 w142 w149 w169 w175 w180 w184 w193 w198 w206 w214 w243 w255 w324 w329 w333 w352 w369 w411 w457 w463 w524 w588 w658 w677 w683 w690 w694 w718 w732]
      tunnel: [w25 w51 w56 w75 w87 w104 w108 w121 w137 w143 w151 w171 w177 w181 w185 w195 w202 w208 w227 w245 w256 w325 w330 w343 w358 w370 w422 w458 w468 w527 w592 w661 w678 w687 w691 w700 w725 w734] -> w14
      tunnel: [_ _ _ _ _ TRUE _ _ _ _ _ _ _ _ _ _ _ _ _ _ _ _ _ _ _ _ _ _ _ _ _ _ _ _ _ _ _ _] -> w13
      tunnel: [w22 w49 w55 w74 w78 w103 w106 w113 w136 w141 w150 w170 w173 w179 w183 w194 w201 w207 w226 w244 w253 w323 w328 w342 w350 w360 w417 w455 w467 w526 w591 w660 w674 w686 w689 w699 w724 w733] -> w12
      tunnel: w10 -> [w21 _ _ _ _ _ _ _ _ _ _ _ _ _ _ _ _ _ _ _ _ _ _ _ _ _ _ _ _ _ _ _ _ _ _ _ _ _]
      frame "", "Event Structure", "Idle" {
        # "executes when the state queue is empty"
        n9 = event shown="[1] \"Exit\": Value Change" {
          selector: _ -> [_ _ _]
          dyn-events: _ -> [_ _ _]
          timeout: w21 -> [_ _ _]
          tunnel: w26 -> [w32 w42 w48]
          tunnel: [w31 w41 w47] -> w25
          tunnel: w24 -> [w29 w39 w45]
          tunnel: [w30 w40 w46] -> w23
          tunnel: w20 -> [w30 w40 w46]
          tunnel: [w29 w39 w45] -> w22
          event Timeout {
            # "Remove Case Structure, as needed."
            # "This is an example of how to enqueue a state periodically. Make sure to set the event structure Timeout >= Period (ms), for this to work."
            # "Timeout Frame\n(this will only execute if the Event Structure timeout is >= 0)"
            n10 = event-data() -> ()  [unwired: 1 in, 1 out]
            n11 = case shown="True" FALSE {
              tunnel: [_ w35] -> w28
              frame False {
              }
              frame True {
                w33 = u32 100  # Period (ms)
                # "Enqueue state periodically"
                n12 = call <vilib>:"Periodic State String__jki_lib_state_machine.vi"("Period (ms)"=w33, "State"="Action: Periodic Work") -> ("State Out"=w35:string)  [unwired: 9 in]
              }
            }
            n13 = call <vilib>:"Add State(s) to Queue__jki_lib_state_machine.vi"("State(s) in Front (\"\")"=w28, "State(s) in (\"\")"=w32) -> ("States Out"=w31:string)  [unwired: 13 in]
          }
          event "Exit": Value Change {
            # "This ensures state is only output if \"OK\" is TRUE. It's not really needed here, since OK has a Latching mechanical action and will reset to FALSE after being read. This merely serves only as an example to show users how one can use Conditional State String."
            # "Exit Button Value Change (pressed) Event\n(this executes Macro: Exit to terminate the VI)"
            n14 = event-data() -> ()  [unwired: 1 in, 1 out]
            n15 = call <vilib>:"Conditional State String__jki_lib_state_machine.vi"("Do State(s)?"="Exit", "State"="Macro: Exit") -> ("State Out"=w36:string)  [unwired: 7 in]
            n16 = call <vilib>:"Add State(s) to Queue__jki_lib_state_machine.vi"("State(s) in Front (\"\")"=w36, "State(s) in (\"\")"=w42) -> ("States Out"=w41:string)  [unwired: 13 in]
          }
          event Panel Close? {
            # "Discard the event because we'll close the front panel ourselves in Macro: Exit"
            # "Close Panel button (pressed) Event\n(this executes Macro: Exit to terminate the VI)"
            n17 = event-data() -> ()  [unwired: 1 in, 1 out]
            n18 = event-data("Discard?"=TRUE) -> ()  [unwired: 1 in, 1 out]
            n19 = call <vilib>:"Add State(s) to Queue__jki_lib_state_machine.vi"("State(s) in Front (\"\")"="Macro: Exit", "State(s) in (\"\")"=w48) -> ("States Out"=w47:string)  [unwired: 13 in]
          }
        }
      }
      frame "---------- Core ----------" {
        # "Do not put any code in this frame.\n(it is a separator no-op)"
        n20 = call <vilib>:"Add State(s) to Queue__jki_lib_state_machine.vi"("State(s) in (\"\")"=w52) -> ("States Out"=w51:string)  [unwired: 14 in]
      }
      frame Default {
        w62 = 42 items=["No error", "Argument error", "Memory is full", "Out of zone", "End of file", "File already open", "Generic file I/O error", "File not found", "File permission error", "Disk is full", "Duplicate path", "Too many files open", "System feature not enabled", "Resource file not found", "Cannot add resource", "Resource not found", "Image not found", "Image memory error", "Pen does not exist", "Config type invalid", "Config token not found", "Config parse error", "Config memory error", "Bad external code format", "Bad external code offset", "External code not present", "Null window", "Destroy window error", "Null menu", "Print aborted", "Bad print record", "Print driver error", "Windows error during printing", "Memory error during printing", "Print dialog error", "Generic print error", "Invalid device refnum", "Device not found", "Device parameter error", "Device unit error", "Cannot open device", "Device call aborted", "Generic error", "Cancelled by user", "Object ID too low", "Object ID too high", "Object not in heap", "Unknown heap", "Unknown object (invalid DefProc)", "Unknown object (DefProc not in table)", "Message out of range", "Invalid (null) method", "Unknown message", "Manager call not supported", "Bad address", "Network operation in progress", "Network operation timed out", "Connection is busy", "Network attribute not supported", "Network error", "Address in use", "System out of memory", "Connection aborted", "Connection refused", "Not connected", "Already connected", "Connection closed", "Initialization error (interapplication manager)", "Bad occurrence", "Wait on unbound occurrence handler", "Occurrence queue overflow", "Datalog type conflict", "Unused", "Unrecognized type (interapplication manager)", "Memory corrupt", "Failed to make temporary DLL", "Old CIN version", "Drag socket not found", "Failed to load drop-object", "Failed to register OLE object", "Failed to release OLE object", "Format specifier type mismatch", "Unknown format specifier", "Too few format specifiers", "Too many format specifiers", "Scan failed", "Newer CIN version", "Error converting to variant", "Runtime menu error", "Password tampered", "Variant attribute not found", "Incompatible variant data type", "Event data is not available", "Event Store is not present", "Occurrence is not found", "Event Queue is not created", "Event info is not available", "Refnum passed is NULL", "Error retrieving Class GUID", "Error retrieving CoClass GUID", "Error retrieving TypeLib GUID.", "Bad built application magic bytes.", "Specific driver is different from the specific driver associated with the Logical Name.", "There is no session opened to the class driver.", "Max Error", "MAX - Error with config objects", "MAX - Error loading configuration", "MAX - Group not supported"]
        # "Current State"
        # "Do not delete, rename, or modify this frame.\n(this is used to capture unhandled states and typos)"
        # "Handle mistyped state name (developer tool)"
        n21 = Format Into String(format string="Software Exception: Unhandled State \"%s\"." ("message"), error in=w58, w53) -> (resulting string=w61:string, error out=w60:errorcluster)  [unwired: 1 in]
        n22 = call <vilib>:"Error Cluster From Error Code.vi"("show call chain? (False)"=TRUE, "error in (no error)"=w60, "error message (\"\")"=w61, "error code (0)"=w62) -> ("error out"=w59:errorcluster)  [unwired: 5 in]
        n23 = call <vilib>:"Add State(s) to Queue__jki_lib_state_machine.vi"("State(s) in (\"\")"=w57) -> ("States Out"=w56:string)  [unwired: 14 in]
      }
      frame "Initialize Core Data" {
        # "Do not delete, rename, or modify this frame.\n(this is used to determine panel behavior on exit)"
        # "originally closed?"
        # "exe?"
        # "If panel starts closed or is an EXE, then close it when we exit"
        n24 = property class="VI"() -> ("FP.State"=w66:T10)  [unwired: 2 in, 2 out]
        n25 = property class="App"() -> ("App.Kind"=w72:T11)  [unwired: 2 in, 2 out]
        n26 = control-ref of="Current VI Reference"() -> (w67:refnum<vi>)
        n27 = Equal?(x=w66, y=T10."Closed" ("Front Panel Window:State")) -> (x = y?=w64:bool)
        n28 = Equal?(x=w72, y=T11."Run Time System" ("Application:Kind")) -> (x = y?=w70:bool)
        n29 = Or(x=w64, y=w70) -> (x .or. y?=w68:bool)
        n30 = Bundle By Name(cluster=w69, "Core.Current VI Reference"=w67, "Core.Close Panel on Exit?"=w68) -> (w74:T13)
        n31 = call <vilib>:"Add State(s) to Queue__jki_lib_state_machine.vi"("State(s) in (\"\")"=w76) -> ("States Out"=w75:string)  [unwired: 14 in]
      }
      frame "Error Handler" {
        # "When running as sourcecode, this function will add previous state data to the error message to aid the developer in troubleshoot errors.\nIf run as an executable, no additional information is added to the error message."
        # "Handle any errors or warnings here.\nYou can also output any states to clean-up after errors or warnings occur"
        # "Clear error or warning"
        n32 = disable-structure shown="Default" {
          disable-tunnel: w85 -> [w99 w100]
          disable-tunnel: w84 -> [w98 _]
          disable-tunnel: [w97 w100] -> w79
          frame condition #0 (active) {
            n33 = call <vilib>:"Append Error Details__jki_lib_state_machine.vi"("error in (no error)"=w99, "Previous State and Argument(s)"=w98) -> ("error out"=w97:errorcluster)  [unwired: 9 in]
          }
          frame condition #1 {
          }
        }
        n34 = Unbundle By Name(w78) -> ("LogFilePath"=w77:path)
        n35 = Unbundle By Name(w79) -> ("code"=w80:i32)
        n36 = case shown="5000..5999" w80 {
          tunnel: w79 -> [_ w92 w96]
          tunnel: w77 -> [_ w91 w93]
          frame 0 {
          }
          frame 5000..5999 {
            n37 = call "ErrorMessage.vi"("error in (no error)"=w92) -> ("Message String"=w89:string)
            n38 = call "WriteLogFile.vi"("Prepend TimeStamp"=FALSE, "Log Message"=w89, "LogFile"=w91) -> ()  [unwired: 8 in, 1 out]
            n39 = invoke on="Messages" class="Str" method="Append String"("string"=w89) -> ()  [unwired: 3 in, 4 out]
          }
          frame Default {
            # "Unhandled Error -- Display it"
            n40 = call <vilib>:"General Error Handler.vi"("error in (no error)"=w96) -> ("message"=w94:string)  [unwired: 10 in, 4 out]
            n41 = call "WriteLogFile.vi"("Prepend TimeStamp"=FALSE, "Log Message"=w94, "LogFile"=w93) -> ()  [unwired: 8 in, 1 out]
          }
        }
        n42 = call-poly <vilib>:"Select State(s)__jki_lib_state_machine.vi"("State(s) if True (\"\")"="Macro: AbortEndOfCycle", "Select"=w79, "State(s) if False (\"\")"="/* Post Warning States") -> ("States Out"=w82:string)  [unwired: 12 in]
        n43 = call <vilib>:"Add State(s) to Queue__jki_lib_state_machine.vi"("State(s) in Front (\"\")"=w82, "State(s) in (\"\")"=w88) -> ("States Out"=w87:string)  [unwired: 13 in]
      }
      frame "Exit" {
        # "Do not put any code in this frame.\n(No errors that occur here will be handled.)"
        n44 = call <vilib>:"Add State(s) to Queue__jki_lib_state_machine.vi"("State(s) in (\"\")"=w105) -> ("States Out"=w104:string)  [unwired: 14 in]
      }
      frame "---------- Data ----------" {
        # "Do not put any code in this frame.\n(It is a separator no-op. You can make a copy of this frame to create a new Data frame)"
        n45 = call <vilib>:"Add State(s) to Queue__jki_lib_state_machine.vi"("State(s) in (\"\")"=w109) -> ("States Out"=w108:string)  [unwired: 14 in]
      }
      frame "Data: Check Folders" {
        # "create top level folder\nif needed"
        n46 = call "MakeTopFolder.vi"("error in (no error)"=w116, "Comment"="Test Name", "Loggers"="Loggers Directory") -> ("error out"=w115:errorcluster, "TopFolderPrefix"=→"TopFolderPrefix":string, "TestFolderPath"=w111:path)  [unwired: 6 in]
        "TopFolderPath" <- w111
        n47 = Build Path(base path=w111, name or relative path="log.txt") -> (appended path=w112:path)
        n48 = Bundle By Name(cluster=w120, "TopFolderPath"=w111, "LogFilePath"=w112) -> (w113:T13)
        n49 = call <vilib>:"Add State(s) to Queue__jki_lib_state_machine.vi"("State(s) in (\"\")"=w122, "State(s) at Back (\"\")"="UI: Status >>Test results Folders OK" ("State(s) at Back (\"\")")) -> ("States Out"=w121:string)  [unwired: 13 in]
      }
      frame "Data: Check Actuation Script" {
        n50 = call <vilib>:"Check if File or Folder Exists.vi"("error in (no error)"=w128, "path"="Path to Actuation Script") -> ("error out"=w130:errorcluster, "file or folder exists?"=w135:bool, "dup path"=w131:path)  [unwired: 7 in]
        n51 = Empty String/Path?(string/path=w131) -> (empty?=w133:bool)
        n52 = Not(x=w133) -> (.not. x?=w134:bool)
        n53 = And(x=w134, y=w135) -> (x .and. y?=w132:bool)
        n54 = Select(t=w130, s=w132, f=errorcluster {"status"=TRUE, "code"=5002, "source"="Actuation Script Not Found"} ("error constant")) -> (s? t:f=w126:errorcluster)
        n55 = Select(t="UI: Status >>Actuation Script Not Found\nUI: Wait for Next1\nData: Check Actuation Script" ("State(s) at Back (\"\")"), s=w126, f="UI: Status >>Actuation Script Found" ("State(s) at Back (\"\")")) -> (s? t:f=w123:string)
        n56 = call <vilib>:"Add State(s) to Queue__jki_lib_state_machine.vi"("State(s) in (\"\")"=w138, "State(s) at Back (\"\")"=w123) -> ("States Out"=w137:string)  [unwired: 13 in]
      }
      frame "Data: Load Definitions" {
        # "load test definitions from file"
        # "Load Test Definitions from File"
        n57 = local read "TestDefinition"() -> (w139:T4)
        n58 = call "Load TestDefinition from XML.vi"("TestDefinition"=w139) -> ("User Specified Out"=w140:T4)  [unwired: 9 in, 1 out]
        n59 = local write "TestDefinition"(w140) -> ()
        n60 = call <vilib>:"Add State(s) to Queue__jki_lib_state_machine.vi"("State(s) in (\"\")"=w144) -> ("States Out"=w143:string)  [unwired: 14 in]
      }
      frame "Data: Review Tests" {
        # "Check Tests"
        n61 = property on="Main Tabs" class="TabCtl (strict)"(error in=w149, "Value"=T1."TestSequence" ("Main Tabs")) -> (error out=w148:errorcluster)  [unwired: 1 in, 1 out]
        n62 = while {
          tunnel: w148 -> [w154]
          tunnel: [w153] -> w147
          stop <- "Next Button 3" stop-if-true
          n63 = Wait Until Next ms Multiple(millisecond multiple=u32 100) -> ()  [unwired: 1 out]
          n64 = case shown="True" "SaveTests" {
            tunnel: [w158 w161] -> w153
            tunnel: w154 -> [w158 w159]
            frame False {
            }
            frame True {
              # "save test definitions to a file"
              n65 = local read "TestDefinition"() -> (w160:T4)
              n66 = call "Save TestDefinition to XML.vi"("error in (no error)"=w159, "TestDefinition"=w160) -> ("error out"=w161:errorcluster)  [unwired: 9 in]
            }
          }
        }
        n67 = call <vilib>:"Add State(s) to Queue__jki_lib_state_machine.vi"("State(s) in (\"\")"=w152, "State(s) at Back (\"\")"="Macro: start tests" ("State(s) at Back (\"\")")) -> ("States Out"=w151:string)  [unwired: 13 in]
      }
      frame "Data: Initialize" {
        w162 = path ""  # LogFilePath
        w163 = T5 {"TTrigger"=-130.0, "Direction"=enum."Falling", "TDelay"=0.0, "Type"=enum."No Test", "Pre-Log (s)"=10.0, "Duration (s)"=30.0, "Post-Log(s)"=100.0}  # CurrentTest
        w164 = 0  # CurrentCycle
        w165 = path ""  # TopFolderPath
        w166 = 0  # TestNumber
        w167 = T14 {"Current VI Reference"=refnum, "Close Panel on Exit?"=FALSE}  # Core
        w168 = ""  # TestPrefix
        # "Data names and types of shift register data are defined by this bundle."
        # "Initialize the shift-register data, here.\n(data names are defined by what you wire into the bundle function)"
        n68 = Bundle("Core"=w167, "CurrentCycle"=w164, "TestNumber"=w166, "TopFolderPath"=w165, "LogFilePath"=w162, "TestPrefix"=w168, "CurrentTest"=w163) -> (w170:T13)  [unwired: 1 in]
        n69 = call <vilib>:"Add State(s) to Queue__jki_lib_state_machine.vi"("State(s) in (\"\")"=w172) -> ("States Out"=w171:string)  [unwired: 14 in]
      }
      frame "Data: Cleanup" {
        # "Cleanup any data and references, here.\n(this is called automatically, by the Macro: Exit)"
        n70 = Unbundle By Name(w173) -> ("Core.Current VI Reference"=w176:refnum<vi>)
        n71 = Close Reference(reference=w176, error in (no error)=w175) -> (error out=w174:errorcluster)
        n72 = call <vilib>:"Add State(s) to Queue__jki_lib_state_machine.vi"("State(s) in (\"\")"=w178) -> ("States Out"=w177:string)  [unwired: 14 in]
      }
      frame "---------- UI ----------" {
        # "Do not put any code in this frame.\n(It is a separator no-op. You can make a copy of this frame to create a new UI frame)"
        n73 = call <vilib>:"Add State(s) to Queue__jki_lib_state_machine.vi"("State(s) in (\"\")"=w182) -> ("States Out"=w181:string)  [unwired: 14 in]
      }
      frame "UI: Wait for Next1" {
        # "Wait for user to press OK button#1"
        n74 = while {
          stop <- "Next1" stop-if-true
          # "Wait for OK button"
        }
        n75 = call <vilib>:"Add State(s) to Queue__jki_lib_state_machine.vi"("State(s) in (\"\")"=w186) -> ("States Out"=w185:string)  [unwired: 14 in]
      }
      frame "UI: Initialize" {
        w188 = ""
        w189 = FALSE ("Heater Enable")
        # "Initialize the User Interface, here.\n(this is called automatically, by the Macro: Initialize)"
        n76 = property on="TED" class="WFChart (strict)"("History Data"=waveform(dbl)[][] []) -> ()  [unwired: 2 in, 2 out]
        n77 = property on="Diode Currents" class="WFChart (strict)"("History Data"=waveform(dbl)[][] []) -> ()  [unwired: 2 in, 2 out]
        n78 = property on="Main Tabs" class="TabCtl (strict)"("Value"=T1."Setup" ("Main Tabs")) -> ()  [unwired: 2 in, 2 out]
        n79 = local write "LED_Illuminate"(w189) -> ()
        n80 = local write "LED_Stimulate"(w189) -> ()
        n81 = local write "PSU Enable"(w189) -> ()
        n82 = local write "Heater Enable"(w189) -> ()
        n83 = call <vilib>:"Add State(s) to Queue__jki_lib_state_machine.vi"("State(s) in (\"\")"=w196) -> ("States Out"=w195:string)  [unwired: 14 in]
        "Status" <- w188
        "Master Logging" <- w189
        "HTR On" <- w189
        "HTR Log" <- w189
        "ACT Logging" <- w189
        "HTR_Fault" <- w189
        "TVC_StopAfterCycle" <- w189
        "ACT Fault" <- w189
        "TEC Fault" <- w189
        "Messages" <- w188
      }
      frame "UI: Uninitialize" {
        w200 = FALSE ("PSU Enable")
        # "Cleanup the User Interface, here.\n(this is called automatically, by the Macro: Exit)"
        n84 = property on="Status" class="Str"(error in=w198, "Value"="Tests Finished" ("Status")) -> (error out=w197:errorcluster)  [unwired: 1 in, 1 out]
        n85 = local write "PSU Enable"(w200) -> ()
        n86 = local write "Master Logging"(w200) -> ()
        n87 = local write "Heater Enable"(w200) -> ()
        n88 = local write "HTR Log"(w200) -> ()
        n89 = local write "ACT Logging"(w200) -> ()
        n90 = call <vilib>:"Add State(s) to Queue__jki_lib_state_machine.vi"("State(s) in (\"\")"=w203) -> ("States Out"=w202:string)  [unwired: 14 in]
      }
      frame "UI: Status" {
        # "Put status information on screen"
        n91 = property on="Status" class="Str"(error in=w206, "Value"=w204) -> (error out=w205:errorcluster)  [unwired: 1 in, 1 out]
        n92 = call <vilib>:"Add State(s) to Queue__jki_lib_state_machine.vi"("State(s) in (\"\")"=w209) -> ("States Out"=w208:string)  [unwired: 14 in]
      }
      frame "UI: Set Datasockets" {
        # "Use control references to point datasocket URLs to local host or TVC machine"
        n93 = control-ref of="TED"() -> (w224:refnum<vi>)
        n94 = control-ref of="Diode Currents"() -> (w212:refnum<vi>)
        n95 = control-ref of="Heater Enable"() -> (w218:refnum<vi>)
        n96 = control-ref of="PSU Enable"() -> (w217:refnum<vi>)
        n97 = control-ref of="LED_Illuminate"() -> (w211:refnum<vi>)
        n98 = control-ref of="LED_Stimulate"() -> (w210:refnum<vi>)
        n99 = control-ref of="TVC_CyclesRemaining"() -> (w219:refnum<vi>)
        n100 = control-ref of="TVC_CycleNumber"() -> (w215:refnum<vi>)
        n101 = control-ref of="TVC_Temperatures"() -> (w220:refnum<vi>)
        n102 = control-ref of="TLUP_Temperatures"() -> (w216:refnum<vi>)
        n103 = control-ref of="Heater Monitor"() -> (w222:refnum<vi>)
        n104 = control-ref of="PSU_Monitor"() -> (w223:refnum<vi>)
        n105 = control-ref of="TEC On"() -> (w225:refnum<vi>)
        n106 = Build Array(w220, w216, w219, w215, w222, w218, w223, w217, w224, w225, w212, w211, w210) -> (w221:refnum<vi>[])
        n107 = for {
          tunnel: w221 -> [w240] mode=indexing
          tunnel: [w231] -> w213
          tunnel: w214 -> [w229]
          # "Use control references to point datasocket URLs to local host or TVC machine"
          n108 = property on="Server IP" class="Ring (strict)"() -> ("RingText.Text"=w239:string)  [unwired: 2 in, 2 out]
          n109 = property class="Ctl"(reference=w240, error in=w229) -> (reference out=w233:refnum<vi>, error out=w230:errorcluster, "DtSktURL"=w236:string)
          n110 = Concatenate Strings("dstp://" ("string"), w239, "/" ("string")) -> (w235:string)
          n111 = call <vilib>:"Search and Replace Pattern.vi"("string"=w236, "regular expression (\"\")"="dstp://.*/" ("regular expression (\"\")"), "replace string (\"\")"=w235) -> ("result string"=w232:string)  [unwired: 2 in, 1 out]
          n112 = property class="Ctl"(reference=w233, error in=w230, "DtSktURL"=w232) -> (error out=w231:errorcluster)  [unwired: 1 out]
        }
        n113 = call <vilib>:"Add State(s) to Queue__jki_lib_state_machine.vi"("State(s) in (\"\")"=w228) -> ("States Out"=w227:string)  [unwired: 14 in]
      }
      frame "UI: Cursor Set" {
        # "Argument"
        # "Set and Unset Cursor Busy.\n(Usage: \"UI: Cursor Set >> Busy|Idle\")"
        n114 = case shown="\"Idle\", Default" w241 {
          tunnel: w243 -> [w248 w250]
          tunnel: [w247 w249] -> w242
          frame "Idle", Default {
            n115 = call <vilib>:"Unset Busy.vi"("error in (no error)"=w248) -> ("error out"=w247:errorcluster)  [unwired: 10 in]
          }
          frame "Busy" {
            n116 = call <vilib>:"Set Busy.vi"("error in (no error)"=w250) -> ("error out"=w249:errorcluster)  [unwired: 9 in, 1 out]
          }
        }
        n117 = call <vilib>:"Add State(s) to Queue__jki_lib_state_machine.vi"("State(s) in (\"\")"=w246) -> ("States Out"=w245:string)  [unwired: 14 in]
      }
      frame "UI: Front Panel State" {
        # "Argument"
        # "Set Front Panel Open or Closed\n(Usage: \"UI: Front Panel State >> Open|Close\")"
        n118 = Unbundle By Name(w253) -> ("Core.Current VI Reference"=w252:refnum<vi>)
        n119 = case shown="\"Minimize\", \"Minimized\"" w251 {
          tunnel: w255 -> [w263 w278 w289 w302 w315]
          tunnel: [w265 w279 w291 w304 w317] -> w254
          tunnel: w252 -> [w264 w276 w290 w303 w316]
          frame "Open", "Standard", Default {
            w258 = T10."Standard" ("State")
            n120 = property class="VI"(reference=w264, error in=w263) -> (reference out=w261:refnum<vi>, error out=w262:errorcluster, "FP.State"=w260:T10)
            n121 = Not Equal?(x=w260, y=w258) -> (x != y?=w259:bool)
            n122 = case shown="True" w259 {
              tunnel: [w269 w271] -> w265
              tunnel: w262 -> [w268 w271]
              tunnel: w261 -> [w267 _]
              tunnel: w258 -> [w266 _]
              frame True {
                n123 = invoke class="VI" method="FP.Open"(reference=w267, error in=w268, "Activate"=TRUE, "State"=w266) -> (error out=w269:errorcluster)  [unwired: 1 in, 4 out]
              }
              frame False {
              }
            }
          }
          frame "Close", "Closed" {
            n124 = property class="VI"(reference=w276, error in=w278) -> (reference out=w275:refnum<vi>, error out=w277:errorcluster, "FP.State"=w273:T10)
            n125 = Not Equal?(x=w273, y=T10."Closed" ("Front Panel Window:State")) -> (x != y?=w272:bool)
            n126 = case shown="True" w272 {
              tunnel: [w280 w283] -> w279
              tunnel: w277 -> [w280 w282]
              tunnel: w275 -> [_ w281]
              frame False {
              }
              frame True {
                n127 = invoke class="VI" method="FP.Close"(reference=w281, error in=w282) -> (error out=w283:errorcluster)  [unwired: 1 in, 2 out]
              }
            }
          }
          frame "Hidden", "Hide" {
            w284 = T10."Hidden" ("State")
            n128 = property class="VI"(reference=w290, error in=w289) -> (reference out=w287:refnum<vi>, error out=w288:errorcluster, "FP.State"=w286:T10)
            n129 = Not Equal?(x=w286, y=w284) -> (x != y?=w285:bool)
            n130 = case shown="True" w285 {
              tunnel: [w295 w296] -> w291
              tunnel: w288 -> [w294 w296]
              tunnel: w287 -> [w293 _]
              tunnel: w284 -> [w292 _]
              frame True {
                n131 = invoke class="VI" method="FP.Open"(reference=w293, error in=w294, "State"=w292) -> (error out=w295:errorcluster)  [unwired: 2 in, 4 out]
              }
              frame False {
              }
            }
          }
          frame "Minimize", "Minimized" {
            w297 = T10."Minimized" ("State")
            n132 = property class="VI"(reference=w303, error in=w302) -> (reference out=w300:refnum<vi>, error out=w301:errorcluster, "FP.State"=w299:T10)
            n133 = Not Equal?(x=w299, y=w297) -> (x != y?=w298:bool)
            n134 = case shown="True" w298 {
              tunnel: [w308 w309] -> w304
              tunnel: w301 -> [w307 w309]
              tunnel: w300 -> [w306 _]
              tunnel: w297 -> [w305 _]
              frame True {
                n135 = invoke class="VI" method="FP.Open"(reference=w306, error in=w307, "State"=w305) -> (error out=w308:errorcluster)  [unwired: 2 in, 4 out]
              }
              frame False {
              }
            }
          }
          frame "Maximize", "Maximized" {
            w310 = T10."Maximized" ("State")
            n136 = property class="VI"(reference=w316, error in=w315) -> (reference out=w313:refnum<vi>, error out=w314:errorcluster, "FP.State"=w312:T10)
            n137 = Not Equal?(x=w312, y=w310) -> (x != y?=w311:bool)
            n138 = case shown="True" w311 {
              tunnel: [w321 w322] -> w317
              tunnel: w314 -> [w320 w322]
              tunnel: w313 -> [w319 _]
              tunnel: w310 -> [w318 _]
              frame True {
                n139 = invoke class="VI" method="FP.Open"(reference=w319, error in=w320, "State"=w318) -> (error out=w321:errorcluster)  [unwired: 2 in, 4 out]
              }
              frame False {
              }
            }
          }
        }
        n140 = call <vilib>:"Add State(s) to Queue__jki_lib_state_machine.vi"("State(s) in (\"\")"=w257) -> ("States Out"=w256:string)  [unwired: 14 in]
      }
      frame "---------- Macro ----------" {
        # "Do not put any code in this frame.\n(It is a separator no-op. You can make a copy of this frame to create a new Macro frame)"
        n141 = call <vilib>:"Add State(s) to Queue__jki_lib_state_machine.vi"("State(s) in (\"\")"=w326) -> ("States Out"=w325:string)  [unwired: 14 in]
      }
      frame "Macro: Initialize" {
        # "Initialization Macro\n(This is called once, when the VI starts)"
        n142 = call <vilib>:"Add State(s) to Queue__jki_lib_state_machine.vi"("State(s) in Front (\"\")"="Data: Initialize\nInitialize Core Data\nUI: Initialize\nUI: Front Panel State >> Open\nUI: Set Datasockets\nData: Load Definitions\nHardware: Setup TVC\nUI: Status >>Setup - Fill in fields and press Next to Continue\nUI: Wait for Next1\nData: Check Folders\nHardware: Check Camera\nUI: Status>> Review Hardware and Press Next to Continue\nHardware: Review\nUI: Status>> Review Test and Press Next to Start Test Sequence\nData: Review Tests ", "State(s) in (\"\")"=w331) -> ("States Out"=w330:string)  [unwired: 13 in]
      }
      frame "Macro: Stabilise" {
        # "stabilise"
        # "Stabilise:\nCall routine to allow system to stabilise"
        n143 = Decimal String To Number(string=w336) -> (number=w335:i32)  [unwired: 2 in, 1 out]
        n144 = property on="Status" class="Str"(error in=w333, "Value"="Stabilisation delay" ("Status")) -> (error out=w334:errorcluster)  [unwired: 1 in, 1 out]
        n145 = control-ref of="DelayRemaining"() -> (w338:refnum<vi>)
        n146 = Multiply(x=60.0 ("y"), y=w335) -> (x*y=w340:dbl)
        n147 = call "DelayTimer.vi"("Formatted \nTime Ref"=w338, "FormatString"="Stabilise: %M:%S", "error in (no error)"=w334, "Delay(s)"=w340) -> ("error out"=w337:errorcluster)  [unwired: 7 in]
        n148 = call <vilib>:"Add State(s) to Queue__jki_lib_state_machine.vi"("State(s) in (\"\")"=w344) -> ("States Out"=w343:string)  [unwired: 14 in]
      }
      frame "Macro: start tests" {
        n149 = property on="Master Logging" class="Bool (strict)"(error in=w352, "Value"=TRUE ("Graphing")) -> (error out=w356:errorcluster)  [unwired: 1 in, 1 out]
        n150 = property on="Temperatures" class="WFChart (strict)"(error in=w356, "History Data"=waveform(dbl)[] []) -> (error out=w355:errorcluster)  [unwired: 1 in, 1 out]
        n151 = Bundle By Name(cluster=w357, "CurrentCycle"=0, "TestNumber"=0 ("CurrentTest")) -> (w350:T13)
        n152 = property on="Main Tabs" class="TabCtl (strict)"(error in=w355, "Value"=T1."Operating" ("Main Tabs")) -> (error out=w351:errorcluster)  [unwired: 1 in, 1 out]
        n153 = call <vilib>:"Add State(s) to Queue__jki_lib_state_machine.vi"("State(s) in (\"\")"=w359, "State(s) at Back (\"\")"="Macro: Wait For Trigger" ("State(s) at Back (\"\")")) -> ("States Out"=w358:string)  [unwired: 13 in]
        "TVC_CyclesRemaining" <- "Cycles To Run"
      }
      frame "Macro: Wait For Trigger" {
        n154 = Unbundle By Name(w361) -> ("TestNumber"=w363:i32)
        n155 = local read "TestDefinition"() -> (w367:T4)
        n156 = Unbundle By Name(w367) -> ("Tests"=w365:T5[])
        n157 = Array Size(array=w365) -> (size(s)=w364:i32)
        n158 = Greater Or Equal?(x=w363, y=w364) -> (x >= y?=w362:bool)
        n159 = case shown="False" w362 {
          tunnel: w369 -> [w384 w406]
          tunnel: [w383 w406] -> w368
          tunnel: [w379 "Macro: End Cycle"] -> w366
          tunnel: w365 -> [w378 _]
          tunnel: w363 -> [w377 _]
          tunnel: w361 -> [w376 w404]
          tunnel: [w375 w404] -> w360
          frame False {
            # "Not at end test yet, so wait for trigger"
            n160 = Index Array(array=w378, index=w377) -> (element=w374:T5)
            n161 = while {
              tunnel: w374 -> [w386]
              tunnel: [w394] -> w381
              tunnel: w384 -> [w391]
              tunnel: [w390] -> w383
              stop <- w397 stop-if-true
              # "Pick temperature reading"
              # "Loop waiting for test condition"
              n162 = local read "TVC_Temperatures"() -> (w387:waveform(dbl)[])
              n163 = Unbundle By Name(w386) -> ("TTrigger"=w393:dbl, "Direction"=w392:enum16{"Rising", "Falling"}, "TDelay"=w394:dbl)
              n164 = Index Array(array=w387, index="ControlChannel") -> (element=w396:waveform(dbl))
              n165 = Unbundle By Name(w396) -> ("Y"=w395:dbl[])
              n166 = Index Array(array=w395) -> (element=w388:dbl)  [unwired: 1 in]
              n167 = call "Make Status Message.vi"("Direction"=w392, "TTrigger"=w393) -> ("Status Message"=w389:string)  [unwired: 9 in]
              n168 = case shown="\"Rising\", Default" w392 {
                tunnel: w388 -> [w399 w402]
                tunnel: w393 -> [w400 w403]
                tunnel: [w398 w401] -> w397
                frame "Rising", Default {
                  # "Trigger when TControl\n>=TTrigger"
                  n169 = Greater Or Equal?(x=w399, y=w400) -> (x >= y?=w398:bool)
                }
                frame "Falling" {
                  # "Trigger when TControl<TTrigger"
                  n170 = Less Or Equal?(x=w402, y=w403) -> (x <= y?=w401:bool)
                }
              }
              n171 = property on="Status" class="Str"(error in=w391, "Value"=w389) -> (error out=w390:errorcluster)  [unwired: 1 in, 1 out]
            }
            n172 = Bundle By Name(cluster=w376, "CurrentTest"=w374) -> (w375:T13)
            n173 = Format Into String(format string="Macro: stabilise>>%d", w381) -> (resulting string=w380:string)  [unwired: 2 in, 1 out]
            n174 = Concatenate Strings(w380, "\r\n", "Macro: Run Test") -> (w379:string)
          }
          frame True {
            # "Tests finished"
          }
        }
        n175 = call <vilib>:"Add State(s) to Queue__jki_lib_state_machine.vi"("State(s) in (\"\")"=w371, "State(s) at Back (\"\")"=w366) -> ("States Out"=w370:string)  [unwired: 13 in]
      }
      frame "Macro: Run Test" {
        n176 = Unbundle By Name(w421) -> ("CurrentTest.Type"=w414:T6, "CurrentTest.TTrigger"=w418:dbl)
        n177 = Not Equal?(x=TestType."No Test", y=w414) -> (x != y?=w419:bool)
        n178 = case shown="True" w419 {
          tunnel: [_ w452] -> w416
          tunnel: [_ w451] -> w415
          tunnel: w418 -> [_ w446]
          frame False {
            # "Don't create directory for null test"
          }
          frame True {
            # "Create Prefix for this test\nand make directory to store \nit in"
            n179 = local read "TopFolderPrefix"() -> (w453:string)
            n180 = local read "TopFolderPath"() -> (w450:path)
            n181 = Add(x="TVC_CycleNumber", y="StartCycle") -> (x+y=w447:i32)
            n182 = call "MakePrefix.vi"("TempPoint"=w446, "TempCycleNo"=w447, "FolderPrefix"=w453, "TopFolderPath"=w450) -> ("Prefix"=w451:string, "TestFolderPath"=w452:path)  [unwired: 6 in]
          }
        }
        n183 = Bundle By Name(cluster=w421, "TopFolderPath"=w416, "TestPrefix"=w415) -> (w417:T13)
        n184 = case shown="\"Diode Test\"" w414 {
          tunnel: "Macro: Run_" -> [w426 w433 w438 w444]
          tunnel: [w427 w431 w439 w445] -> w412
          tunnel: ["" w429 w435 w441] -> w408
          tunnel: "Preparing" -> [_ w428 w434 w440]
          frame "No Test", Default {
            n185 = Concatenate Strings(w426, "NULL" ("string")) -> (w427:string)
          }
          frame "Heater Test" {
            n186 = Concatenate Strings(w428, " Heater " ("string")) -> (w429:string)
            n187 = Concatenate Strings(w433, "HTR" ("string")) -> (w431:string)
          }
          frame "Actuation Test" {
            n188 = Concatenate Strings(w434, " Actuation " ("string")) -> (w435:string)
            n189 = Concatenate Strings(w438, "ACT" ("string")) -> (w439:string)
          }
          frame "Diode Test" {
            n190 = Concatenate Strings(w440, " Diode " ("string")) -> (w441:string)
            n191 = Concatenate Strings(w444, "DIODE" ("string")) -> (w445:string)
          }
        }
        n192 = Concatenate Strings(w408, "Test" ("string")) -> (w410:string)
        n193 = property on="Status" class="Str"("Value"=w410) -> ()  [unwired: 2 in, 2 out]
        n194 = call <vilib>:"Add State(s) to Queue__jki_lib_state_machine.vi"("State(s) in (\"\")"=w423, "State(s) at Back (\"\")"=w412) -> ("States Out"=w422:string)  [unwired: 13 in]
      }
      frame "Macro: Run_NULL" {
        # "NULL Test - Does nothing except increment test numbe and go back\nto wait for trigger"
        n195 = in-place {
          n196 = in-place-cluster #1(w456) -> ("TestNumber"=w461:i32)
          n197 = Increment(x=w461) -> (x+1=w460:i32)
          n198 = in-place-cluster #1("TestNumber"=w460) -> (w455:T13)
        }
        n199 = call <vilib>:"Add State(s) to Queue__jki_lib_state_machine.vi"("State(s) in (\"\")"=w459, "State(s) at Back (\"\")"="Macro: Wait For Trigger" ("State(s) at Back (\"\")")) -> ("States Out"=w458:string)  [unwired: 13 in]
      }
      frame "Macro: Run_HTR" {
        # "Heater Test"
        n200 = local read "HTR_Fault"() -> (w462:bool)
        n201 = case shown="False" w462 {
          tunnel: w465 -> [w495 _]
          tunnel: [w475 w518] -> w464
          tunnel: w463 -> [w471 w518]
          frame False {
            # "Form heater log names"
            n202 = Unbundle By Name(w495) -> ("TopFolderPath"=w494:path, "TestPrefix"=w493:string, "CurrentTest"=w489:T5, "LogFilePath"=w473:path)
            n203 = local read "TestDefinition"() -> (w492:T4)
            n204 = call "WriteLogFile.vi"("error in (no error)"=w471, "Log Message"="Start Heater Test", "LogFile"=w473) -> ("error out"=w470:errorcluster)  [unwired: 8 in]
            n205 = Unbundle By Name(w492) -> ("PSU  Log Period (ms)"=w502:i64, "Temperature Log Period(ms)"=w503:i64)
            n206 = property on="HTR Log" class="Bool (strict)"(error in=w470, "Value"=TRUE ("Heater Logging")) -> (error out=w476:errorcluster)  [unwired: 1 in, 1 out]
            n207 = Concatenate Strings(w493, "Temp.xlsx" ("string")) -> (w499:string)
            n208 = Concatenate Strings(w493, "PSU.xlsx" ("string")) -> (w500:string)
            n209 = Build Path(base path=w494, name or relative path=w499) -> (appended path=w498:path)
            n210 = Build Path(base path=w494, name or relative path=w500) -> (appended path=w501:path)
            n211 = while {
              tunnel: w501 -> [w515]
              tunnel: w502 -> [w511]
              tunnel: w476 -> [_]
              stop <- w512 stop-if-true
              n212 = Wait Until Next ms Multiple(millisecond multiple=w511) -> ()  [unwired: 1 out]
              n213 = local read "Heater Monitor"() -> (w514:waveform(dbl)[])
              n214 = local read "PSU_Monitor"() -> (w513:waveform(dbl)[])
              n215 = local read "HTR Log"() -> (w517:bool)
              n216 = Not(x=w517) -> (.not. x?=w512:bool)
              n217 = Merge Signals(w514, w513) -> (w516:dynamicdata)
              n218 = call "Write Voltage and Current Log File"("Signals"=w516, "Flush? (T)"=w512, "Filename"=w515) -> ()  [unwired: 14 in, 3 out]
            }
            n219 = while {
              tunnel: w498 -> [w510]
              tunnel: w503 -> [w504]
              tunnel: w476 -> [_]
              stop <- w508 stop-if-true
              n220 = local read "TLUP_Temperatures"() -> (w506:waveform(dbl)[])
              n221 = local read "TVC_Temperatures"() -> (w507:waveform(dbl)[])
              n222 = Wait Until Next ms Multiple(millisecond multiple=w504) -> ()  [unwired: 1 out]
              n223 = local read "HTR Log"() -> (w505:bool)
              n224 = Not(x=w505) -> (.not. x?=w508:bool)
              n225 = Merge Signals(w507, w506) -> (w509:dynamicdata)
              n226 = call "Write Temperature Log File"("Signals"=w509, "Flush? (T)"=w508, "Filename"=w510) -> ()  [unwired: 14 in, 3 out]
            }
            n227 = control-ref of="Heater Monitor"() -> (w478:refnum<vi>)
            n228 = control-ref of="HTR Log"() -> (w479:refnum<vi>)
            n229 = control-ref of="HTR_Fault"() -> (w482:refnum<vi>)
            n230 = control-ref of="Status"() -> (w490:refnum<vi>)
            n231 = control-ref of="DelayRemaining"() -> (w491:refnum<vi>)
            n232 = control-ref of="HTR On"() -> (w480:refnum<vi>)
            n233 = control-ref of="HTR_Fault"() -> (w481:refnum<vi>)
            n234 = call "HTR_Check.vi"("HTR_Fault ref"=w481, "HTR ON Ref"=w480, "Logging Ref"=w479, "error in (no error)"=w476, "HTR_Monitor Ref"=w478, "Heater Test Options"="Heater Test Options") -> ("error out"=w474:errorcluster)  [unwired: 5 in]
            n235 = control-ref of="HTR On"() -> (w483:refnum<vi>)
            n236 = control-ref of="Heater Enable"() -> (w488:refnum<vi>)
            n237 = call "HTR_Test.vi"("HTR_Enable Ref"=w488, "HTR_OnOff Ref"=w483, "DelayRemaining"=w491, "Status Ref"=w490, "error in (no error)"=w476, "Abort Ref"=w482, "CurrentTest"=w489) -> ("error out"=w484:errorcluster)  [unwired: 4 in]
            n238 = property on="HTR Log" class="Bool (strict)"(error in=w484, "Value"=FALSE ("Heater Logging")) -> (error out=w485:errorcluster)  [unwired: 1 in, 1 out]
            n239 = Merge Errors(w474, w485) -> (w475:errorcluster)
          }
          frame True {
          }
        }
        n240 = in-place {
          n241 = in-place-cluster #2(w465) -> ("TestNumber"=w520:i32)
          n242 = Increment(x=w520) -> (x+1=w519:i32)
          n243 = in-place-cluster #2("TestNumber"=w519) -> (w467:T13)
        }
        n244 = call <vilib>:"Add State(s) to Queue__jki_lib_state_machine.vi"("State(s) in (\"\")"=w469, "State(s) at Back (\"\")"="Macro: Wait For Trigger" ("State(s) at Back (\"\")")) -> ("States Out"=w468:string)  [unwired: 13 in]
      }
      frame "Macro: Run_DIODE" {
        # "Run Diode Test"
        n245 = local read "TEC Fault"() -> (w521:bool)
        n246 = case shown="False" w521 {
          tunnel: w524 -> [w555 w583]
          tunnel: w523 -> [w554 _]
          tunnel: [w536 w583] -> w522
          frame False {
            w532 = "Diode Test Start" ("Status")
            # "Wait a sec"
            # "Form Diode log names"
            # "Start Logging before \nenabling Peltier"
            n247 = Unbundle By Name(w554) -> ("TopFolderPath"=w552:path, "TestPrefix"=w553:string)
            n248 = Unbundle By Name(w554) -> ("CurrentTest"=w530:T5, "LogFilePath"=w531:path)
            n249 = property on="Status" class="Str"(error in=w555, "Value"=w532) -> (error out=w533:errorcluster)  [unwired: 1 in, 1 out]
            n250 = local read "TestDefinition"() -> (w551:T4)
            n251 = call "WriteLogFile.vi"("error in (no error)"=w533, "Log Message"=w532, "LogFile"=w531) -> ("error out"=w534:errorcluster)  [unwired: 8 in]
            n252 = Unbundle By Name(w530) -> ("Pre-Log (s)"=w529:dbl)
            n253 = Unbundle By Name(w551) -> ("Temperature Log Period(ms)"=w562:i64)
            n254 = property on="Diode Logging" class="Bool (strict)"(error in=w534, "Value"=TRUE ("Heater PSU")) -> (error out=w550:errorcluster)  [unwired: 1 in, 1 out]
            n255 = Concatenate Strings(w553, "Diode.xlsx" ("string")) -> (w560:string)
            n256 = call <userlib>:"Wait (ms)__ogtk.vi"("error in (no error)"=w550, "milliseconds to wait"=u32 1000) -> ("error out"=w539:errorcluster)  [unwired: 8 in, 1 out]
            n257 = Build Path(base path=w552, name or relative path=w560) -> (appended path=w559:path)
            n258 = control-ref of="DelayRemaining"() -> (w546:refnum<vi>)
            n259 = Multiply(x=w529, y=1000.0) -> (x*y=w540:dbl)
            n260 = control-ref of="TEC Fault"() -> (w537:refnum<vi>)
            n261 = call <userlib>:"Wait (ms)__ogtk.vi"("error in (no error)"=w539, "milliseconds to wait"=w540) -> ("error out"=w538:errorcluster)  [unwired: 8 in, 1 out]
            n262 = while {
              tunnel: w559 -> [w582]
              tunnel: w550 -> [_]
              tunnel: w562 -> [w576]
              stop <- w580 stop-if-true
              n263 = Wait Until Next ms Multiple(millisecond multiple=w576) -> ()  [unwired: 1 out]
              n264 = local read "Diode Logging"() -> (w577:bool)
              n265 = local read "TLUP_Temperatures"() -> (w578:waveform(dbl)[])
              n266 = local read "TVC_Temperatures"() -> (w579:waveform(dbl)[])
              n267 = local read "Diode Currents"() -> (w575:waveform(dbl)[])
              n268 = local read "TED"() -> (w574:waveform(dbl)[])
              n269 = Not(x=w577) -> (.not. x?=w580:bool)
              n270 = Merge Signals(w574, w575, w579, w578) -> (w581:dynamicdata)
              n271 = call "Write Diode Log File"("Signals"=w581, "Flush? (T)"=w580, "Filename"=w582) -> ()  [unwired: 14 in, 3 out]
            }
            n272 = while {
              tunnel: "Diode Test Options" -> [w573]
              tunnel: w538 -> [w569]
              tunnel: [w568] -> w535
              stop <- w566 stop-if-true
              # "Check for Abort conditions"
              n273 = local read "TED Status"() -> (w571:T3[])
              n274 = local read "Diode Logging"() -> (w567:bool)
              n275 = local read "Diode Currents"() -> (w570:waveform(dbl)[])
              n276 = local read "LED_Stimulate"() -> (w572:bool)
              n277 = Not(x=w567) -> (.not. x?=w565:bool)
              n278 = call "Diode_Check.vi"("Stim.On?"=w572, "error in (no error)"=w569, "Diode Currents"=w570, "TED Status"=w571, "Diode Test Options"=w573) -> ("error out"=w568:errorcluster, "TEC Fault"=w564:bool)  [unwired: 5 in]
              n279 = Or(x=w564, y=w565) -> (x .or. y?=w566:bool)
              n280 = local write "TEC Fault"(w564) -> ()
              n281 = Wait Until Next ms Multiple(millisecond multiple=u32 200) -> ()  [unwired: 1 out]
            }
            n282 = control-ref of="TEC On"() -> (w548:refnum<vi>)
            n283 = control-ref of="LED_Stimulate"() -> (w547:refnum<vi>)
            n284 = call "DiodeTest.vi"("Stimulus_LED"=w547, "Peltier_OnOffs"=w548, "DelayStr Ref"=w546, "Abort Ref"=w537, "error in (no error)"=w539, "CurrentTest"=w530) -> ("error out"=w561:errorcluster)  [unwired: 5 in]
            n285 = property on="Diode Logging" class="Bool (strict)"(error in=w561, "Value"=FALSE ("Heater Logging")) -> (error out=w545:errorcluster)  [unwired: 1 in, 1 out]
            n286 = property on="Status" class="Str"(error in=w545, "Value"="Diode Test Finish" ("Status")) -> (error out=w544:errorcluster)  [unwired: 1 in, 1 out]
            n287 = Merge Errors(w535, w544) -> (w536:errorcluster)
          }
          frame True {
          }
        }
        n288 = in-place {
          n289 = in-place-cluster #3(w523) -> ("TestNumber"=w585:i32)
          n290 = Increment(x=w585) -> (x+1=w584:i32)
          n291 = in-place-cluster #3("TestNumber"=w584) -> (w526:T13)
        }
        n292 = call <vilib>:"Add State(s) to Queue__jki_lib_state_machine.vi"("State(s) in (\"\")"=w528, "State(s) at Back (\"\")"="Macro: Wait For Trigger" ("State(s) at Back (\"\")")) -> ("States Out"=w527:string)  [unwired: 13 in]
      }
      frame "Macro: Run_ACT" {
        # "ACT Test - Runs actuation test"
        n293 = local read "ACT Fault"() -> (w586:bool)
        n294 = case shown="False" w586 {
          tunnel: w589 -> [w607 _]
          tunnel: w588 -> [w603 w649]
          tunnel: [w601 w649] -> w587
          frame False {
            w594 = TRUE ("LED_Illuminate")
            w598 = "Actuation Test" ("Status")
            # "Test storage Directory"
            # "TestPrefix"
            n295 = property on="Status" class="Str"(error in=w603, "Value"=w598) -> (error out=w599:errorcluster)  [unwired: 1 in, 1 out]
            n296 = Unbundle By Name(w607) -> ("TopFolderPath"=w605:path, "TestPrefix"=w606:string, "CurrentTest"=w602:T5, "LogFilePath"=w597:path)
            n297 = local read "TestDefinition"() -> (w604:T4)
            n298 = call "WriteLogFile.vi"("error in (no error)"=w599, "Log Message"=w598, "LogFile"=w597) -> ("error out"=w600:errorcluster)  [unwired: 8 in]
            n299 = Unbundle By Name(w604) -> ("ActuationsPerLoop"=w608:i32)
            n300 = property on="LED_Illuminate" class="Bool (strict)"(error in=w600, "Value"=w594) -> (error out=w595:errorcluster)  [unwired: 1 in, 1 out]
            n301 = property on="PSU Enable" class="Bool (strict)"(error in=w595, "Value"=w594) -> (error out=w596:errorcluster)  [unwired: 1 in, 1 out]
            n302 = for {
              N: w608 -> [_]
              shift-right: [w611] -> w601
              shift-left: w596 -> [w620]
              tunnel: w604 -> [w624]
              tunnel: w606 -> [w623]
              tunnel: w605 -> [w622]
              tunnel: w602 -> [w612]
              i -> [w633]
              stop <- w611 stop-if-true
              # "Add Actuation\nto TestPrefix"
              n303 = Format Into String(format string="A%d_", initial string=w623, w633) -> (resulting string=w613:string)  [unwired: 1 in, 1 out]
              n304 = property on="ACT Logging" class="Bool (strict)"(error in=w620, "Value"=TRUE ("Actuation Logging")) -> (error out=w619:errorcluster)  [unwired: 1 in, 1 out]
              n305 = Unbundle By Name(w624) -> ("PSU  Log Period (ms)"=w626:i64, "Temperature Log Period(ms)"=w625:i64)
              n306 = Concatenate Strings(w613, "PSU.xlsx" ("string")) -> (w630:string)
              n307 = Build Path(base path=w622, name or relative path=w630) -> (appended path=w629:path)
              n308 = local read "Camera"() -> (w615:string)
              n309 = control-ref of="DelayRemaining"() -> (w618:refnum<vi>)
              n310 = Concatenate Strings(w613, "Temp.xlsx" ("string")) -> (w632:string)
              n311 = local read "Path to Actuation Script"() -> (w616:path)
              n312 = Build Path(base path=w622, name or relative path=w632) -> (appended path=w631:path)
              n313 = while {
                tunnel: w631 -> [w643]
                tunnel: w619 -> [_]
                tunnel: w625 -> [w637]
                stop <- w641 stop-if-true
                # "write log file, \nbuffer to memory\nflush on exit"
                # "write Temperature log"
                n314 = Wait Until Next ms Multiple(millisecond multiple=w637) -> ()  [unwired: 1 out]
                n315 = local read "TLUP_Temperatures"() -> (w638:waveform(dbl)[])
                n316 = local read "TVC_Temperatures"() -> (w639:waveform(dbl)[])
                n317 = local read "ACT Logging"() -> (w640:bool)
                n318 = Not(x=w640) -> (.not. x?=w641:bool)
                n319 = Merge Signals(w639, w638) -> (w642:dynamicdata)
                n320 = call "Write Actuation Temperature Log"("Signals"=w642, "Flush? (T)"=w641, "Filename"=w643) -> ()  [unwired: 14 in, 3 out]
              }
              n321 = while {
                tunnel: w629 -> [w647]
                tunnel: w619 -> [_]
                tunnel: w626 -> [w644]
                stop <- w645 stop-if-true
                # "write log file, \nbuffer to memory\nflush on exit"
                # "write Board PSU log"
                n322 = Wait Until Next ms Multiple(millisecond multiple=w644) -> ()  [unwired: 1 out]
                n323 = local read "ACT Logging"() -> (w646:bool)
                n324 = local read "PSU_Monitor"() -> (w648:waveform(dbl)[])
                n325 = Not(x=w646) -> (.not. x?=w645:bool)
                n326 = call "Write Actuation PSU Log"("Signals"=w648, "Flush? (T)"=w645, "Filename"=w647) -> ()  [unwired: 14 in, 3 out]
              }
              n327 = local read "FFMPEG exe"() -> (w617:path)
              n328 = call "ACT_Test.vi"("COM Port"="COM Port", "Path to FFMPEG"=w617, "Video Camera"=w615, "Path to Actuation Script"=w616, "error in (no error)"=w619, "Test Prefix"=w613, "DelayStr Ref"=w618, "CurrentTest"=w612) -> ("error out"=w611:errorcluster)  [unwired: 3 in]
              n329 = case shown="Error .." w611 {
                frame No Error {
                }
                frame Error {
                  n330 = local write "ACT Fault"(TRUE ("ACT Fault")) -> ()
                }
              }
              n331 = flat-sequence {
                tunnel: w611 -> [_]
                tunnel: w611 -> [_]
                frame #0 {
                  n332 = property on="ACT Logging" class="Bool (strict)"("Value"=FALSE ("Actuation Logging")) -> ()  [unwired: 2 in, 2 out]
                }
              }
            }
            n333 = flat-sequence {
              tunnel: w601 -> [_]
              frame #0 {
                n334 = property on="LED_Illuminate" class="Bool (strict)"("Value"=FALSE ("LED_Illuminate")) -> ()  [unwired: 2 in, 2 out]
                n335 = property on="PSU Enable" class="Bool (strict)"("Value"=FALSE ("PSU Enable")) -> ()  [unwired: 2 in, 2 out]
              }
            }
          }
          frame True {
          }
        }
        n336 = in-place {
          n337 = in-place-cluster #4(w589) -> ("TestNumber"=w651:i32)
          n338 = Increment(x=w651) -> (x+1=w650:i32)
          n339 = in-place-cluster #4("TestNumber"=w650) -> (w591:T13)
        }
        n340 = call <vilib>:"Add State(s) to Queue__jki_lib_state_machine.vi"("State(s) in (\"\")"=w593, "State(s) at Back (\"\")"="Macro: Wait For Trigger" ("State(s) at Back (\"\")")) -> ("States Out"=w592:string)  [unwired: 13 in]
      }
      frame "Macro: End Cycle" {
        n341 = Unbundle By Name(w655) -> ("CurrentCycle"=w654:i32, "LogFilePath"=w656:path)
        n342 = in-place {
          in-place-border: [w663] -> w659
          n343 = in-place-cluster #5(w655) -> ("CurrentCycle"=w668:i32)  [unwired: 1 out]
          n344 = Increment(x=w668) -> (x+1=w664:i32)
          n345 = local read "Cycles To Run"() -> (w667:i32)
          n346 = Greater Or Equal?(x=w664, y=w667) -> (x >= y?=w666:bool)
          n347 = case shown="False" w666 {
            tunnel: [0 _] -> w665
            tunnel: ["Macro: Wait For Trigger" "Macro: Exit"] -> w663
            frame False {
            }
            frame True {
            }
          }
          n348 = in-place-cluster #5("CurrentCycle"=w664, "TestNumber"=w665) -> (w660:T13)
        }
        n349 = Format Into String(format string="Test Cycle %d finished" ("Log Message"), w654) -> (resulting string=w652:string)  [unwired: 2 in, 1 out]
        n350 = call "WriteLogFile.vi"("error in (no error)"=w658, "Log Message"=w652, "LogFile"=w656) -> ("error out"=w657:errorcluster)  [unwired: 8 in]
        n351 = call <vilib>:"Add State(s) to Queue__jki_lib_state_machine.vi"("State(s) in (\"\")"=w662, "State(s) at Back (\"\")"=w659) -> ("States Out"=w661:string)  [unwired: 13 in]
      }
      frame "Macro: AbortEndOfCycle" {
        n352 = Unbundle By Name(w674) -> ("LogFilePath"=w675:path)
        n353 = call "WriteLogFile.vi"("error in (no error)"=w677, "Log Message"="Aborting at end of TVC Cycle", "LogFile"=w675) -> ("error out"=w676:errorcluster)  [unwired: 8 in]
        n354 = local write "TVC_StopAfterCycle"(TRUE ("TVC_StopAfterCycle")) -> ()
        n355 = call <vilib>:"Add State(s) to Queue__jki_lib_state_machine.vi"("State(s) in (\"\")"=w679) -> ("States Out"=w678:string)  [unwired: 14 in]
      }
      frame "Macro: Exit" {
        # "Exit Macro\n(This is called once, when the VI exits)"
        n356 = Unbundle By Name(w686) -> ("Core.Close Panel on Exit?"=w681:bool)
        n357 = call <vilib>:"Conditional State String__jki_lib_state_machine.vi"("Do State(s)?"=w681, "State"="UI: Front Panel State >> Close") -> ("State Out"=w680:string)  [unwired: 7 in]
        n358 = call <vilib>:"Add State(s) to Queue__jki_lib_state_machine.vi"("State(s) in (\"\")"=w680, "State(s) at Back (\"\")"="UI: Uninitialize\nData: Cleanup\nExit") -> ("States Out"=w684:string)  [unwired: 13 in]
        n359 = call <vilib>:"Add State(s) to Queue__jki_lib_state_machine.vi"("State(s) in Front (\"\")"=w684, "State(s) in (\"\")"=w688) -> ("States Out"=w687:string)  [unwired: 13 in]
      }
      frame "---------- Hardware ----------" {
        # "Template Separator\n(You can make a copy of, or modify, this frame)"
        n360 = call <vilib>:"Add State(s) to Queue__jki_lib_state_machine.vi"("State(s) in (\"\")"=w692) -> ("States Out"=w691:string)  [unwired: 14 in]
      }
      frame "Hardware: Setup TVC" {
        n361 = while {
          tunnel: ["TVC_Temperatures"] -> w696
          tunnel: [w708] -> w698
          tunnel: w694 -> [w707]
          stop <- w710 stop-if-true
          # "Wait Until TVC Temperatures connected"
          n362 = property on="TVC_Temperatures" class="Arr (strict)"(error in=w707) -> (error out=w708:errorcluster, "DtSktStatus"=w713:T15)  [unwired: 1 in, 1 out]
          n363 = Unbundle By Name(w713) -> ("Code"=w712:T12)
          n364 = Equal?(x=w712, y=T12."Active") -> (x = y?=w710:bool)
        }
        n365 = for {
          tunnel: w696 -> [w706] mode=indexing
          tunnel: "NI_ChannelName" ("name") -> [w705]
          tunnel: [w704] -> w697 mode=indexing
          tunnel: w698 -> [w703]
          tunnel: [w702] -> w693
          n366 = Get Waveform Attribute(4:w703, 5:w705, 6:w705, 7:w706) -> (0:w702:errorcluster, 1:w704:string)  [unwired: 2 out]
        }
        "ChannelNames" <- w697
        n367 = property on="ControlChannel" class="Ring (strict)"("Strings []"=w697) -> ()  [unwired: 2 in, 2 out]
        n368 = call <vilib>:"Add State(s) to Queue__jki_lib_state_machine.vi"("State(s) in (\"\")"=w701) -> ("States Out"=w700:string)  [unwired: 14 in]
      }
      frame "Hardware: Check Camera" {
        # "check FFMPeg exists"
        n369 = call <vilib>:"Check if File or Folder Exists.vi"("error in (no error)"=w718, "path"="FFMPEG exe") -> ("error out"=w721:errorcluster, "file or folder exists?"=w722:bool)  [unwired: 7 in, 1 out]
        n370 = Select(t=w721, s=w722, f=errorcluster {"status"=TRUE, "code"=5001, "source"="Video Device Not Found"} ("error constant")) -> (s? t:f=w720:errorcluster)
        n371 = call "FindVideoDevices.vi"("error in (no error)"=w720, "Path to FFMPEG"="FFMPEG exe") -> ("error out"=w716:errorcluster, "Video Devices"=w723:string[])  [unwired: 8 in]
        n372 = property on="Video Camera" class="Ring (strict)"("Strings []"=w723) -> ()  [unwired: 2 in, 2 out]
        n373 = property on="Status" class="Str"(error in=w716, "Value"="Camera OK" ("State(s) at Back (\"\")")) -> (error out=w715:errorcluster)  [unwired: 1 in, 1 out]
        n374 = call <vilib>:"Add State(s) to Queue__jki_lib_state_machine.vi"("State(s) in (\"\")"=w726) -> ("States Out"=w725:string)  [unwired: 14 in]
      }
      frame "Hardware: Review" {
        # "save text from Video Camera \ncontrol to pass into capture routine"
        n375 = property on="Main Tabs" class="TabCtl (strict)"(error in=w732, "Value"=T1."Hardware" ("Main Tabs")) -> (error out=w731:errorcluster)  [unwired: 1 in, 1 out]
        n376 = while {
          tunnel: w731 -> [w737]
          tunnel: [w737] -> w729
          stop <- "Next2" stop-if-true
          n377 = Wait Until Next ms Multiple(millisecond multiple=u32 100) -> ()  [unwired: 1 out]
        }
        n378 = property on="Video Camera" class="Ring (strict)"(error in=w729) -> (error out=w728:errorcluster, "RingText.Text"=→"Camera":string)  [unwired: 1 in, 1 out]
        n379 = call <vilib>:"Add State(s) to Queue__jki_lib_state_machine.vi"("State(s) in (\"\")"=w735) -> ("States Out"=w734:string)  [unwired: 14 in]
      }
    }
  }
  n380 = case shown="True" w4 {
    frame False {
    }
    frame True {
      n381 = local read "TestDefinition"() -> (w740:T4)
      n382 = Unbundle By Name(w740) -> ("Temperature Log Period(ms)"=w741:i64)
      n383 = while {
        tunnel: w741 -> [w755]
        stop <- w758 continue-if-true
        # "draw graph of  Temperatures"
        n384 = local read "TLUP_Temperatures"() -> (w756:waveform(dbl)[])
        n385 = local read "TVC_Temperatures"() -> (w752:waveform(dbl)[])
        n386 = Wait Until Next ms Multiple(millisecond multiple=w755) -> ()  [unwired: 1 out]
        n387 = local read "ControlChannel"() -> (w750:u16)
        n388 = local read "Master Logging"() -> (w758:bool)
        n389 = Merge Signals(w752, w756) -> (→"Temperatures":dynamicdata)
        n390 = Index Array(array=w752, index=w750) -> (element=w753:waveform(dbl))
        n391 = Unbundle By Name(w753) -> ("Y"=w754:dbl[])
        n392 = Index Array(array=w754) -> (element=→"Trigger Point Reading":dbl)  [unwired: 1 in]
      }
      n393 = local read "TopFolderPrefix"() -> (w744:string)
      n394 = local read "TopFolderPath"() -> (w745:path)
      n395 = Concatenate Strings(w744, "_Temp.xlsx") -> (w749:string)
      n396 = Build Path(base path=w745, name or relative path=w749) -> (appended path=w748:path)
      n397 = while {
        tunnel: w748 -> [w770]
        tunnel: w741 -> [w764]
        i -> [w762]
        stop <- w768 stop-if-true
        # "write Temperature log\nwrite log file, buffer to memory\nflush on exit or every 100 readings"
        n398 = local read "Master Logging"() -> (w767:bool)
        n399 = Wait Until Next ms Multiple(millisecond multiple=w764) -> ()  [unwired: 1 out]
        n400 = local read "TLUP_Temperatures"() -> (w765:waveform(dbl)[])
        n401 = local read "TVC_Temperatures"() -> (w766:waveform(dbl)[])
        n402 = Quotient & Remainder(x=w762, y=100) -> (x-y*floor(x/y)=w760:i32)  [unwired: 1 out]
        n403 = Not(x=w767) -> (.not. x?=w768:bool)
        n404 = Equal To 0?(x=w760) -> (x = 0?=w759:bool)
        n405 = Or(x=w768, y=w759) -> (x .or. y?=w763:bool)
        n406 = Merge Signals(w766, w765) -> (w769:dynamicdata)
        n407 = call "Write Master Temperature"("Signals"=w769, "Flush? (T)"=w763, "Filename"=w770) -> ()  [unwired: 14 in, 3 out]
      }
      n408 = Unbundle By Name(w740) -> ("PSU  Log Period (ms)"=w739:i64)
      n409 = Concatenate Strings(w744, "_PSU.xlsx") -> (w747:string)
      n410 = Build Path(base path=w745, name or relative path=w747) -> (appended path=w746:path)
      n411 = while {
        tunnel: w746 -> [w781]
        tunnel: w739 -> [w779]
        i -> [w772]
        stop <- w773 stop-if-true
        # "write Board PSU log\nwrite log file, buffer to memory\nflush on exit or every 100 readings"
        n412 = Wait Until Next ms Multiple(millisecond multiple=w779) -> ()  [unwired: 1 out]
        n413 = local read "Master Logging"() -> (w780:bool)
        n414 = local read "Heater Monitor"() -> (w777:waveform(dbl)[])
        n415 = local read "PSU_Monitor"() -> (w782:waveform(dbl)[])
        n416 = Quotient & Remainder(x=w772, y=1000) -> (x-y*floor(x/y)=w775:i32)  [unwired: 1 out]
        n417 = Not(x=w780) -> (.not. x?=w773:bool)
        n418 = Equal To 0?(x=w775) -> (x = 0?=w776:bool)
        n419 = Merge Signals(w777, w782) -> (w778:dynamicdata)
        n420 = Or(x=w773, y=w776) -> (x .or. y?=w771:bool)
        n421 = call "Write Master PSU Log"("Signals"=w778, "Flush? (T)"=w771, "Filename"=w781) -> ()  [unwired: 14 in, 3 out]
      }
    }
  }
